vi "SynthHD_3_2a.vi"() -> ()   [LabVIEW 2017]
uses:
  Tab1.ctl
  <vilib>/Utility/file.llb/Write Delimited Spreadsheet (DBL).vi
  <vilib>/Utility/file.llb/Read Delimited Spreadsheet (DBL).vi
panel:
  in  "boot":bool=TRUE
  out "HD2":bool
  in  "CSD":bool
  out "RFOnB2":bool
  out "RFOnA2":bool
  out "Level B 2":bool
  out "Level A 2":bool
  in  "Modon":bool
  in  "Sync":bool
  out "POWER dBm B":dbl min=-100.0 max=24.0 step=1.0 format="%.2g"
  out "POWER dBm A":dbl min=-100.0 max=24.0 step=1.0 format="%.2g"
  out "RF  FREQUENCY MHz  B":dbl=1000.0 min=54.0 max=13900.0 step=1.0 format="%.7g"
  out "RF  FREQUENCY MHz A":dbl=1000.0 min=54.0 max=13900.0 step=1.0 format="%.7g"
  out "Amp Delta A -B":dbl format="%.2g"
  out "Freq Delta A-B":dbl format="%.7f"
  out "Device Under Control":string
  in  "AKNR":bool
  in  "PKNR":bool
  in  "FKNR":bool
  out "Channel":string="A"
  in  "ChSt":bool=TRUE
  out "COM Error":bool
  in  "Serial Port Select":refnum<visa-resource-name>="COM3"
  in  "stop":bool
  in  "Main Tab":T1
  in  "adn":bool
  in  "aup":bool
  in  "pdn":bool
  in  "pup":bool
  in  "fdn":bool
  in  "fup":bool
  out "Level":bool
  in  "Power Step Size":i32(ring)=3 items=["0.01dB", "0.05dB", "0.1 dB", "0.5 dB", "1.0 dB", "5.0 dB", "10.0 dB"]
  in  "RF  FREQUENCY MHz":dbl=1000.0 min=53.0 max=13999.999 step=1.0 format="%.7g"
  in  "Freqkn":i8(knob)=1 scale=1.0..20.0
  in  "Phasekn":i8(knob)=1 scale=1.0..20.0
  in  "PHASE Degrees":dbl min=0.0 max=360.0 step=1.0 format="%.2g"
  in  "POWER dBm":dbl min=-75.0 max=20.0 step=1.0 format="%.2g"
  in  "Powerkn":i8(knob)=1 scale=1.0..20.0
  in  "Frequency Step Size":i32(ring)=7 items=["0.1Hz", "1Hz", "10Hz", "100Hz", "1KHz", "10KHz", "100KHz", "1MHz", "10MHz", "100MHz", "1GHz"]
  in  "Phase Step Size":i32(ring)=6 items=["0.01 Degree", "0.05 Degree", "0.1 Degree", "0.5 Degree", "1 Degree", "5 Degree", "10 Degree", "90 Degree", "180 Degree"]
  in  "RF On":bool=TRUE
  in  "ChLock":bool
  in  "Sweep":enum32{"Linear", "List"}(tab)
  in  "Leveling":bool
  in  "Start Frequency":dbl=54.0 min=53.0 max=13999.999 step=0.001 format="%7.7f"
  in  "Step Size MHz (or %)":dbl=50.0 min=1e-07 max=23990.0 step=0.001 format="%.7f"
  in  "Stop Frequency":dbl=4000.0 min=53.0 max=13999.999 step=0.001 format="%7.7f"
  in  "Start Amplitude":dbl=22.0 min=-80.0 max=22.0 step=0.01 format="%7.2f"
  in  "Stop Amplitude":dbl=22.0 min=-80.0 max=22.0 step=0.01 format="%7.2f"
  out "Number\nof Points":u16
  out "Time per\nSweep (mS)":dbl format="%#.6g"
  in  "SwType":bool
  in  "Read Table\nFrom  CSV":bool
  in  "Save Table\nTo CSV File":bool
  in  "Table RAM to\nTable NVROM":bool
  in  "Send Table\nTo RAM":bool
  in  "Sweep Table":dbl[][](array[numeric]) format="%#.6f"
  in  "Read Table\nFrom Device":bool
  in  "sweepdiff":bool
  in  "Sweep\nOnce":bool
  in  "Sweep\nContinuously":bool
  in  "sweepdir":bool
  in  "Differential Freq":dbl=54.0 min=-13800.0 max=13800.0 step=0.001 format="%7.7f"
  in  "Step Time (mS)":dbl=4.0 min=0.1 max=10000.0 step=0.001 format="%.3f"
  out "Swpc":string
  in  "Mod Tab":enum32{"PULSE Amplitude", "AM", "FM"}(tab)
  in  "Dual Channel Mode":bool
  in  "Send Pulse\nBurst":bool
  out "Duration (uS)":dbl
  in  "Continuous\nPM":bool
  in  "# of Pulses in Burst":u16=100 min=1 max=65500 step=1 format="%#.5f"
  in  "Off Time (uS)":u32=10 min=2 max=10000000 step=1
  in  "On Time (uS)":u32=1 max=10000000 step=1
  out "Pulsech":string
  in  "Invert\nPulse":bool
  in  "Read AM":bool
  out "Samples/Cycle":u8
  in  "Save AM to ROM":bool
  out "AMch":string
  in  "AM Freq (Hz)":dbl=500.0 min=1.0 max=5000.0 step=1.0 format="%.2f"
  out "Actual Freq (Hz)":dbl
  in  "Peak Power(dBm)":dbl=15.0 min=-74.9 max=20.0 step=0.01 format="%.2f"
  in  "Minimum Power (dBm)":dbl=15.0 min=-74.9 max=20.0 step=0.01 format="%.2f"
  in  "Continuous AM":bool
  in  "Wave Shape":u8(ring) items=["Sine", "Ramp", "Triangle"]
  out "Waveform":dbl[](graph)
  in  "Linear in?":u8(ring) items=["Linear in dB", "Linear in Volts"]
  in  "AM Samples in Burst":u16=100 min=1 max=5000 step=1 format="%#.5f"
  in  "FM Rate (Hz)":u16=500 min=1 max=20000 step=1
  in  "FM Deviation (+/- Hz)":u32=500 min=10 step=1
  in  "Continuous FM":bool
  in  "FM Samples in Burst":u16=100 min=1 max=65500 step=1 format="%#.5f"
  out "FMch":string
  in  "FM Function":u8(ring) items=["Sine", "Chirp"]
  out "FM Samples / Cycle":u16
  out "Specific Instructions":string
  in  "Trigger":i32(ring) items=["No Triggers", "Full Frequency Sweep", "Single Sweep Step", "Stop All", "Digital RF On/Off", "Remove Interrupts", "Reserved 1", "Reserved 2", "Ext AM Modulation", "Ext FM Modulation"]
  out "read buffer":string
  in  "Query1":bool
  in  "Query2":bool
  in  "Query3":bool
  in  "Query4":bool
  in  "MUX Out Select":u8(ring)=6 items=["HiZ", "Vdd", "GND", "R Divider", "N Divider", "An Lock Det", "Dig Lock Det"]
  in  "PLL ICP":u8=4 max=15 step=1 format="%02d"
  out "HW Version":string
  in  "Get Phase\nLock Status":bool
  out "FW Version":string
  in  "Read\nVersion":bool
  in  "Save Settings\nto ROM":bool
  in  "Get\nTemperature":bool
  out "Temperature":string
  in  "Fundamental\nFeedback Mode":bool
  out "Lock":bool
  in  "MTLD":bool
  in  "Re-Init Settings\nto Default":bool
  in  "Reference Select":u8(ring)=1 items=["External", "Internal 27MHz", "Internal 10MHz"]
  in  "Reference (MHz)":dbl=27.0 min=5.0 max=111.0 step=0.001 format="%7.6g"
  in  "AutoCal":bool=TRUE
  in  "Channel\nSpacing":dbl=100.0 min=0.01 max=10000.0 step=0.01 format="%.2f"
  # "A"
  # "B"
  # "v3.2a"
  # "Windfreak Technologies"
  # "A"
  # "B"
  # "Tab selection dictates sweep mode"
  # "Step"
  # "Freq(MHz)"
  # "Level(dBm)"
  # "right click table for more options"
  # "Burst"
  # "Software will not respond during \"Pulse Burst\" for lower jitter."
  # "Widest FM Deviation+/- \n54-106.25MHz = 160KHz\n-212.5MHz        = 312KHz\n-425.0MHz        = 625KHz\n-850.0MHz      = 1.25MHz\n-1700MHz         = 2.5MHz\n-3400MHz            = 5MHz\n-6800MHz          = 10MHz\n-13600MHz        = 20MHz"
  # "Digital Trigger 0V to +3.3V only.\nAnalog Input 0V to 1.2V only.\nTrigger has ~35K ohm pullup\nfor both modes."
  # "Read Settings"
  # "C"
  # "Windfreak Technologies, LLC 2019"
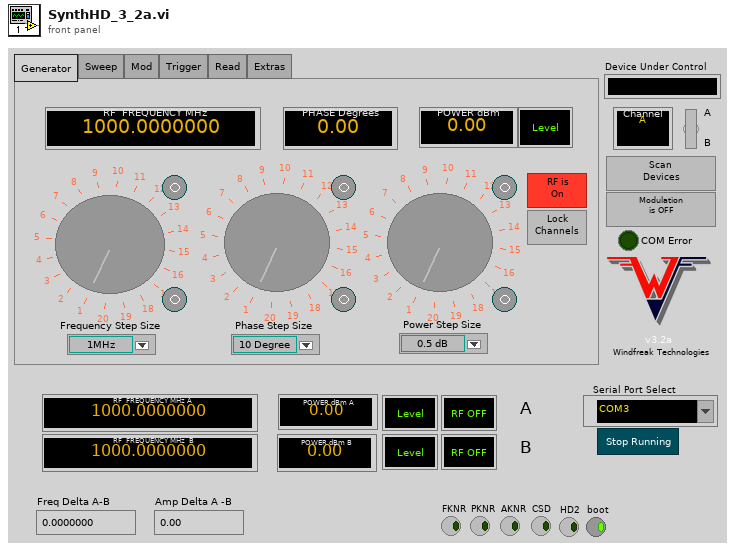
[diagram p1: front panel]
types:
  T1 = typedef "Tab1.ctl" = enum32{"Generator", "Sweep", "Mod", "Trigger", "Read", "Extras"}
  T2 = enum8{"Enabled", "Disabled", "Disabled and Grayed Out"}
  T3 = cluster{"[0]":dbl, "[1]":dbl, "[2]":dbl, "[3]":dbl, "[4]":dbl, "[5]":dbl, "[6]":dbl, "[7]":dbl, "[8]":dbl, "[9]":dbl, "[10]":dbl, "[11]":dbl, "[12]":dbl, "[13]":dbl, "[14]":dbl, "[15]":dbl, "[16]":dbl, "[17]":dbl, "[18]":dbl, "[19]":dbl, "[20]":dbl, "[21]":dbl, "[22]":dbl, "[23]":dbl, "[24]":dbl, "[25]":dbl, "[26]":dbl, "[27]":dbl, "[28]":dbl, "[29]":dbl, "[30]":dbl, "[31]":dbl, "[32]":dbl, "[33]":dbl, "[34]":dbl, "[35]":dbl, "[36]":dbl, "[37]":dbl, "[38]":dbl, "[39]":dbl, "[40]":dbl, "[41]":dbl, "[42]":dbl, "[43]":dbl, "[44]":dbl}
  T4 = typedef "LVPoint32TypeDef.ctl" = cluster{"Horizontal":i32, "Vertical":i32}
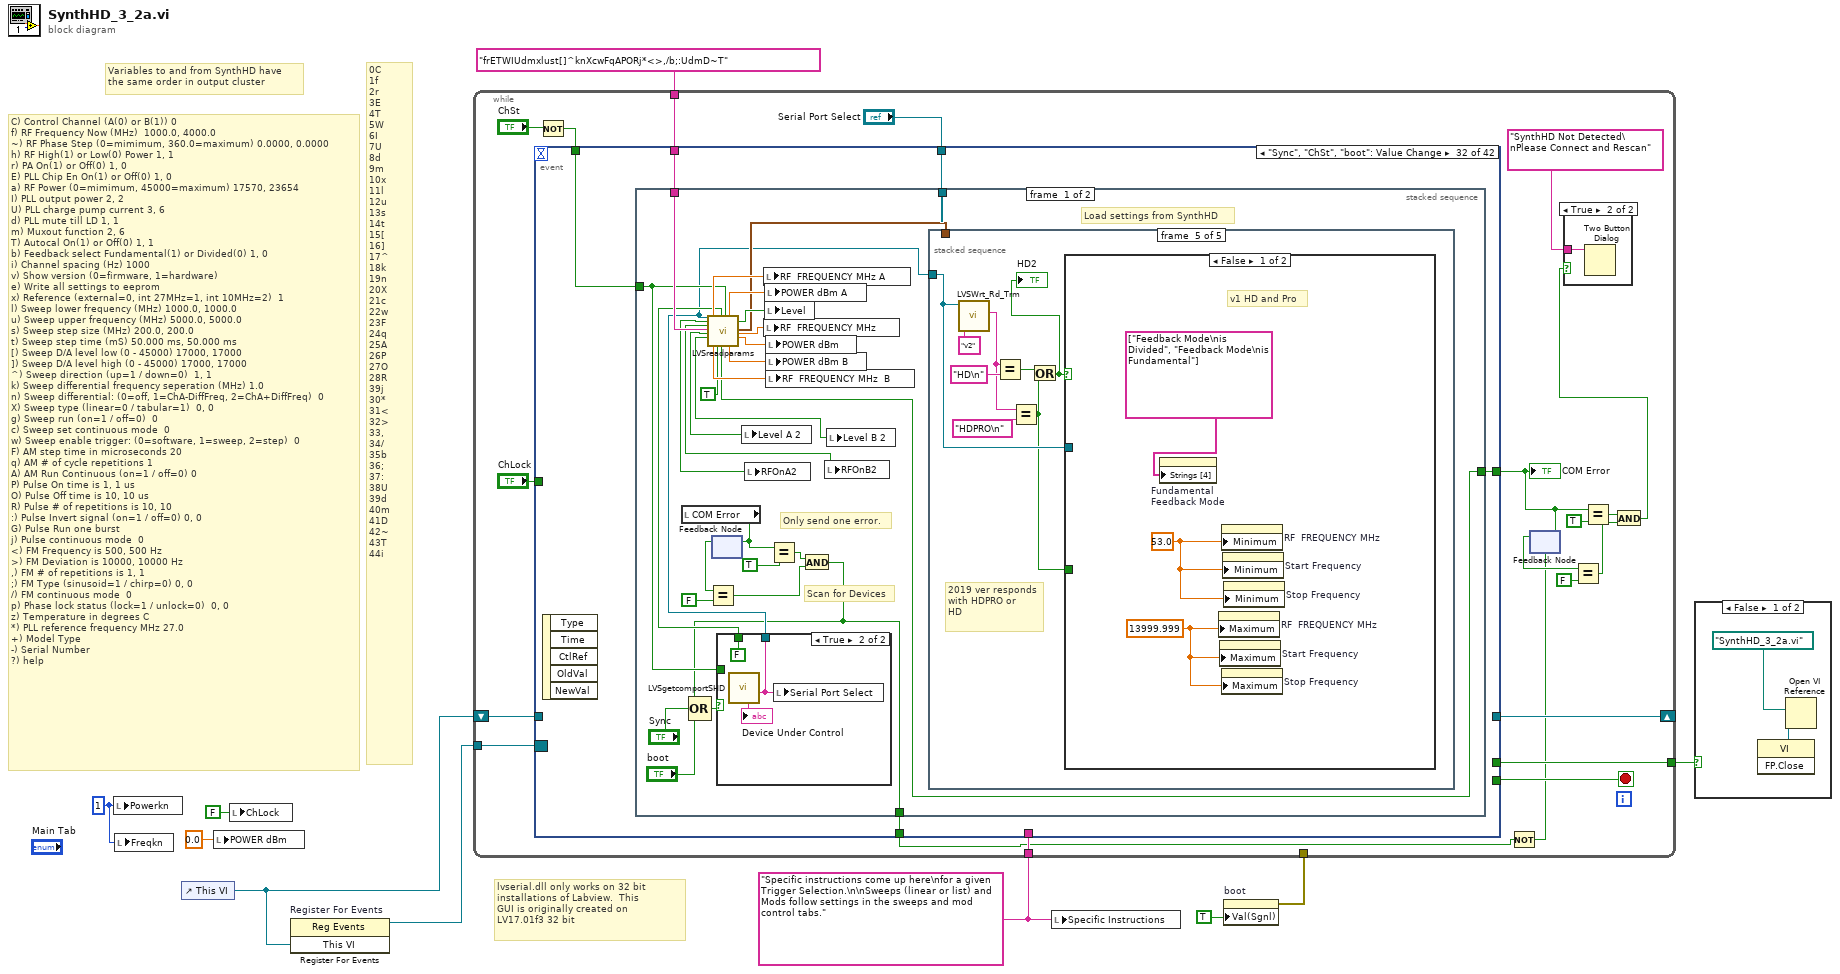
[diagram p0: block diagram]
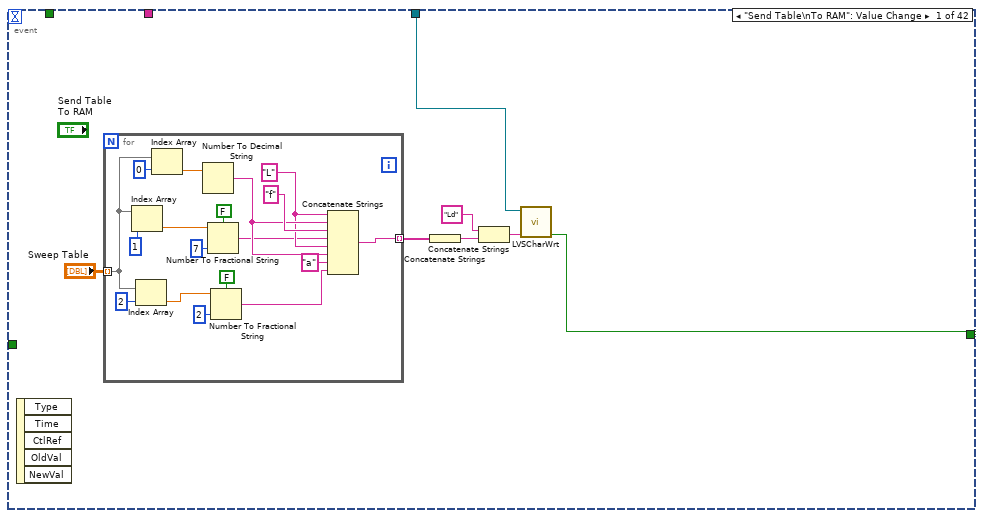
[diagram p4: hidden frame]
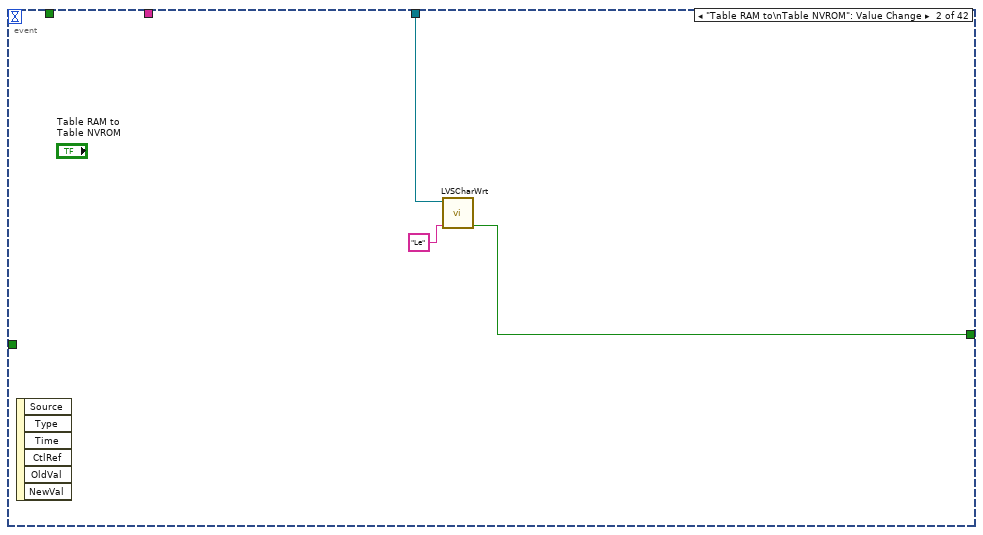
[diagram p5: hidden frame]
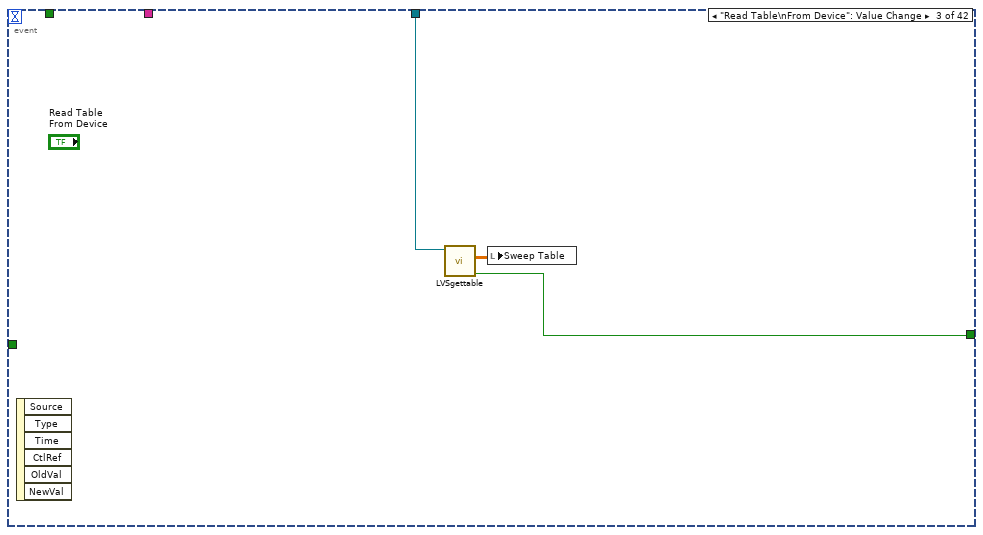
[diagram p6: hidden frame]
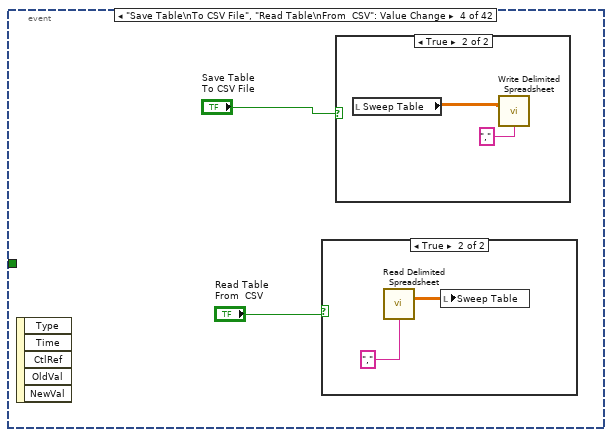
[diagram p7: hidden frame]
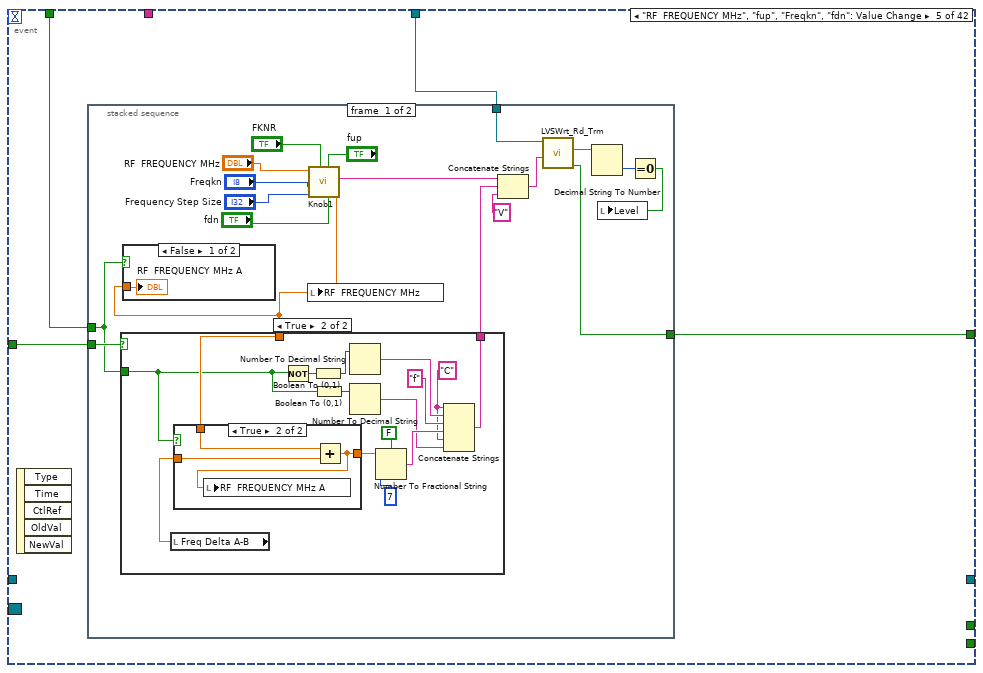
[diagram p10: hidden frame]
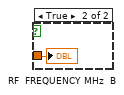
[diagram p11: hidden frame]
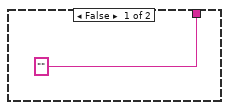
[diagram p12: hidden frame]
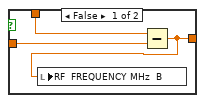
[diagram p13: hidden frame]
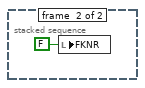
[diagram p14: hidden frame]
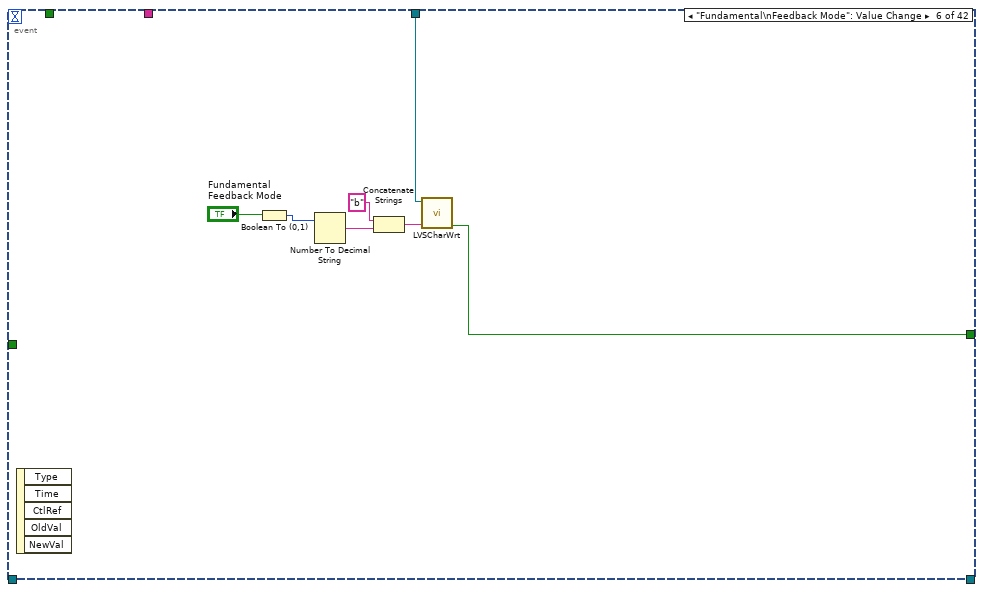
[diagram p15: hidden frame]
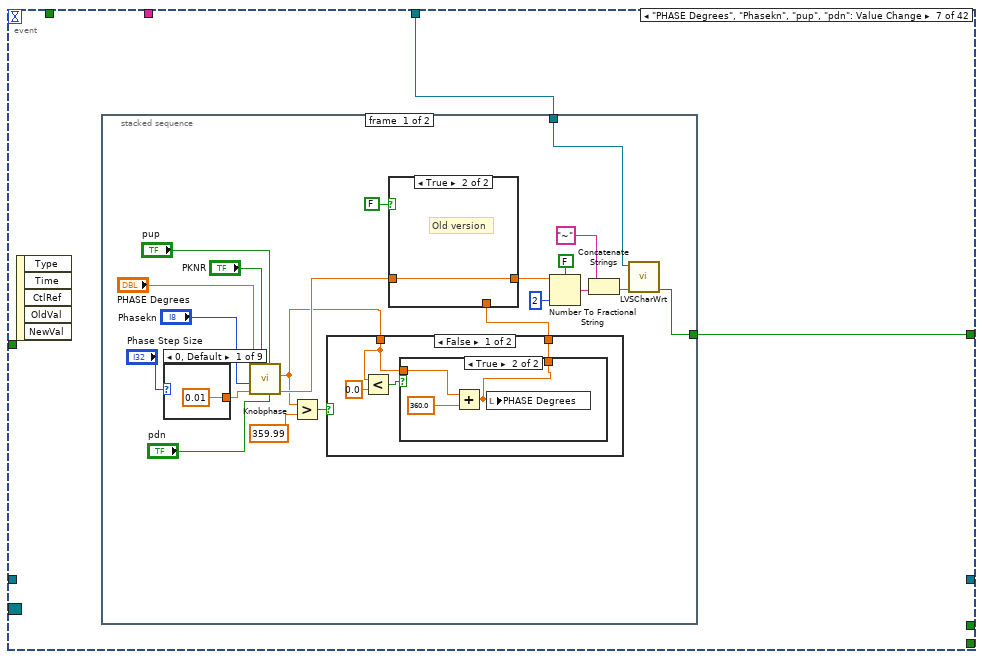
[diagram p16: hidden frame]
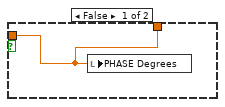
[diagram p18: hidden frame]
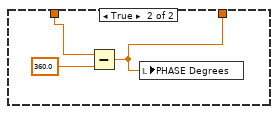
[diagram p19: hidden frame]
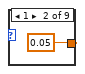
[diagram p20: hidden frame]
diagram:
  w4 = "Specific instructions come up here\nfor a given Trigger Selection.\n\nSweeps (linear or list) and Mods follow settings in the sweeps and mod control tabs." ("message")
  w8 = i8 1 ("Powerkn")
  # "lvserial.dll only works on 32 bit\ninstallations of Labview.  This\nGUI is originally created on\nLV17.01f3 32 bit"
  # "C) Control Channel (A(0) or B(1)) 0\nf) RF Frequency Now (MHz)  1000.0, 4000.0\n~) RF Phase Step (0=mimimum, 360.0=maximum) 0.0000, 0.0000\nh) RF High(1) or Low(0) Power 1, 1\nr) PA On(1) or Off(0) 1, 0\nE) PLL Chip En On(1) or Off(0) 1, 0\na) RF Power (0=mimimum, 45000=maximum) 17570, 23654\nI) PLL output power 2, 2\nU) PLL charge pump current 3, 6\nd) PLL mute till LD 1, 1\nm) Muxout function 2, 6\nT) Autocal On(1) or Off(0) 1, 1\nb) Feedback select Fundamental(1) or Divided(0) 1, 0\ni) Channel spacing (Hz) 1000\nv) Show version (0=firmware, 1=hardware)\ne) Write all settings to eeprom\nx) Reference (external=0, int 27MHz=1, int 10MHz=2)  1\nl) Sweep lower frequency (MHz) 1000.0, 1000.0\nu) Sweep upper frequency (MHz) 5000.0, 5000.0\ns) Sweep step size (MHz) 200.0, 200.0\nt) Sweep step time (mS) 50.000 ms, 50.000 ms\n[) Sweep D/A level low (0 - 45000) 17000, 17000\n]) Sweep D/A level high (0 - 45000) 17000, 17000\n^) Sweep direction (up=1 / down=0)  1, 1\nk) Sweep differential frequency seperation (MHz) 1.0\nn) Sweep differential: (0=off, 1=ChA-DiffFreq, 2=ChA+DiffFreq)  0\nX) Sweep type (linear=0 / tabular=1)  0, 0\ng) Sweep run (on=1 / off=0)  0\nc) Sweep set continuous mode  0\nw) Sweep enable trigger: (0=software, 1=sweep, 2=step)  0\nF) AM step time in microseconds 20\nq) AM # of cycle repetitions 1\nA) AM Run Continuous (on=1 / off=0) 0\nP) Pulse On time is 1, 1 us\nO) Pulse Off time is 10, 10 us\nR) Pulse # of repetitions is 10, 10\n:) Pulse Invert signal (on=1 / off=0) 0, 0\nG) Pulse Run one burst\nj) Pulse continuous mode  0\n<) FM Frequency is 500, 500 Hz\n>) FM Deviation is 10000, 10000 Hz\n,) FM # of repetitions is 1, 1\n;) FM Type (sinusoid=1 / chirp=0) 0, 0\n/) FM continuous mode  0\np) Phase lock status (lock=1 / unlock=0)  0, 0\nz) Temperature in degrees C\n*) PLL reference frequency MHz 27.0\n+) Model Type\n-) Serial Number  \n?) help"
  # "0C\n1f\n2r\n3E\n4T\n5W\n6I\n7U\n8d\n9m\n10x\n11l\n12u\n13s\n14t\n15[\n16]\n17^\n18k\n19n\n20X\n21c\n22w\n23F\n24q\n25A\n26P\n27O\n28R\n39j\n30*\n31<\n32>\n33,\n34/\n35b\n36;\n37:\n38U\n39d\n40m\n41D\n42~\n43T\n44i"
  # "Variables to and from SynthHD have \nthe same order in output cluster"
  n1 = local write "Powerkn"(w8) -> ()
  n2 = local write "Freqkn"(w8) -> ()
  n3 = control-ref of="This VI"() -> (w6:refnum<vi>)
  n4 = local write "POWER dBm"(0.0 ("Power")) -> ()
  n5 = local write "ChLock"(FALSE ("ChLock")) -> ()
  n6 = register-events "Register For Events"(w6) -> (reference out=w7:refnum<event-registration>)  [unwired: 2 in, 1 out]
  n7 = local write "Specific Instructions"(w4) -> ()
  n8 = property on="boot" class="Bool (strict)"("Val(Sgnl)"=TRUE ("boot")) -> (error out=w2:errorcluster)  [unwired: 2 in, 1 out]
  n9 = while {
    shift-right: [w27] -> _
    shift-left: w6 -> [w29]
    tunnel: w7 -> [w28]
    tunnel: [w26] -> w5
    tunnel: "frETWIUdmxlust[]^knXcwFqAPORj*<>,/b;:UdmD~T" ("var query") -> [w25]
    tunnel: w4 -> [w21]
    tunnel: w2 -> [_]
    stop <- w30 stop-if-true
    n10 = Not(x="ChSt") -> (.not. x?=w23:bool)
    n11 = event shown="[31] \"Sync\", \"ChSt\", \"boot\": Value Change" {
      selector: w28 -> [_ _ _ _ _ _ _ _ _ _ _ _ _ _ _ _ _ _ _ _ _ _ _ _ _ _ _ _ _ _ _ _ _ _ _ _ _ _ _ _ _ _]
      dyn-events: _ -> [_ _ _ _ _ _ _ _ _ _ _ _ _ _ _ _ _ _ _ _ _ _ _ _ _ _ _ _ _ _ _ _ _ _ _ _ _ _ _ _ _ _]
      timeout: _ -> [_ _ _ _ _ _ _ _ _ _ _ _ _ _ _ _ _ _ _ _ _ _ _ _ _ _ _ _ _ _ _ _ _ _ _ _ _ _ _ _ _ _]
      tunnel: "Serial Port Select" -> [w33 w59 w62 _ w73 w118 w125 w173 w238 _ w266 w317 w327 w344 w362 w387 w406 w409 w439 w442 w461 w471 w474 w481 w486 w495 w498 w516 w523 w530 w541 w552 w712 w720 w748 w766 _ _ _ _ w858 w870]
      tunnel: [_ _ _ _ _ _ _ _ _ _ _ _ _ _ _ _ _ _ _ _ _ _ _ _ _ _ _ _ _ _ _ _ _ _ _ _ _ "stop" w854 _ _ _] -> w30
      tunnel: w29 -> [_ _ _ _ _ _ _ _ _ _ _ _ _ _ _ _ _ _ _ _ _ _ _ _ _ _ _ _ _ _ _ _ _ _ _ _ _ _ w853 _ _ _]
      tunnel: [_ _ _ _ _ _ _ _ _ _ _ _ _ _ _ _ _ _ _ _ _ _ _ _ _ _ _ _ _ _ _ _ _ _ _ _ _ _ w853 _ _ _] -> w27
      tunnel: [_ _ _ _ _ _ _ _ _ _ _ _ _ _ _ _ _ _ _ _ _ _ _ _ _ _ _ _ _ _ _ _ _ _ _ _ _ "stop" _ _ _ _] -> w26
      tunnel: w25 -> [_ _ _ _ _ _ _ _ _ _ _ _ _ _ _ _ _ _ _ _ _ _ _ _ _ _ _ _ _ _ _ w553 _ _ _ _ _ _ _ _ _ _]
      tunnel: w23 -> [_ _ _ _ w72 _ _ w172 w241 _ _ _ _ _ w363 w394 _ w420 _ w449 _ _ _ _ _ _ _ _ _ _ _ w551 _ _ w752 _ _ _ _ _ _ _]
      tunnel: "ChLock" -> [_ _ _ _ w71 _ _ w171 _ _ _ _ _ _ _ _ _ _ _ _ _ _ _ _ _ _ _ _ _ _ _ _ _ _ _ _ _ _ _ _ _ _]
      tunnel: w21 -> [_ _ _ _ _ _ _ _ _ _ _ _ w329 _ _ _ _ _ _ _ _ _ _ _ _ _ _ _ _ _ _ _ _ _ _ _ _ _ _ _ _ _]
      tunnel: [w34 w58 w61 _ w70 w117 w124 w170 w237 _ w263 w316 w326 w343 w361 w386 w405 w408 w437 w440 w459 w470 w473 w479 w482 w492 w496 w515 w521 w528 w540 w550 w711 w719 w747 w765 w785 _ _ _ w857 _] -> w15
      tunnel: [_ _ _ _ _ _ _ _ _ _ _ _ _ _ _ _ _ _ _ _ _ _ _ _ _ _ _ _ _ _ _ w549 _ _ _ _ _ _ _ _ _ _] -> w12
      event "Send Table\nTo RAM": Value Change {
        n12 = event-data() -> ()  [unwired: 1 in, 5 out]
        n13 = for {
          tunnel: "Sweep Table" -> [w46] mode=indexing
          tunnel: [w52] -> w36 mode=indexing
          w49 = "L" ("string")
          n14 = Index Array(array=w46, index=1) -> (element=w45:dbl)
          n15 = Index Array(array=w46, index=2) -> (element=w41:dbl)
          n16 = Index Array(array=w46, index=0) -> (element=w50:dbl)
          n17 = Number To Decimal String(number=w50) -> (decimal integer string=w53:string)  [unwired: 1 in]
          n18 = Number To Fractional String(use system decimal point (T)=FALSE, number=w45, precision (6)=i16 7) -> (F-format string=w48:string)  [unwired: 1 in]
          n19 = Number To Fractional String(use system decimal point (T)=FALSE, number=w41, precision (6)=i16 2) -> (F-format string=w40:string)  [unwired: 1 in]
          n20 = Concatenate Strings(w49, w53, "f" ("string"), w48, w49, w53, "a" ("string"), w40) -> (w52:string)
        }
        n21 = Concatenate Strings(w36) -> (w38:string)
        n22 = Concatenate Strings("Ld" ("string"), w38) -> (w35:string)
        n23 = call "LVSCharWrt.vi"("String In"=w35, "COM Port"=w33) -> ("ComError"=w34:bool)  [unwired: 9 in]
      }
      event "Table RAM to\nTable NVROM": Value Change {
        n24 = event-data() -> ()  [unwired: 1 in, 6 out]
        n25 = call "LVSCharWrt.vi"("String In"="Le" ("write buffer"), "COM Port"=w59) -> ("ComError"=w58:bool)  [unwired: 9 in]
      }
      event "Read Table\nFrom Device": Value Change {
        n26 = event-data() -> ()  [unwired: 1 in, 6 out]
        n27 = call "LVSgettable.vi"("Serial Port Select"=w62) -> ("COM Error"=w61:bool, "Sweep Table"=w63:dbl[][])  [unwired: 9 in]
        n28 = local write "Sweep Table"(w63) -> ()
      }
      event "Save Table\nTo CSV File", "Read Table\nFrom  CSV": Value Change {
        n29 = event-data() -> ()  [unwired: 1 in, 5 out]
        n30 = case shown="True" "Read Table\nFrom  CSV" {
          frame False {
          }
          frame True {
            n31 = call-poly <vilib>:"Read Delimited Spreadsheet.vi"("delimiter (\\t)"="," ("delimiter (\\t)")) -> ("all rows"=w67:dbl[][])  [unwired: 9 in, 5 out]
            n32 = local write "Sweep Table"(w67) -> ()
          }
        }
        n33 = case shown="True" "Save Table\nTo CSV File" {
          frame False {
          }
          frame True {
            n34 = local read "Sweep Table"() -> (w69:dbl[][])
            n35 = call-poly <vilib>:"Write Delimited Spreadsheet.vi"("2D data"=w69, "delimiter (\\t)"="," ("delimiter (\\t)")) -> ()  [unwired: 12 in, 2 out]
          }
        }
      }
      event "RF  FREQUENCY MHz", "fup", "Freqkn", "fdn": Value Change {
        n36 = event-data() -> ()  [unwired: 1 in, 5 out]
        n37 = stacked-sequence {
          tunnel: w73 -> [w77 _]
          tunnel: w72 -> [w82 _]
          tunnel: w71 -> [w84 _]
          tunnel: [w75 _] -> w70
          frame #0 {
            n38 = call "Knob1.vi"("Freqin"="RF  FREQUENCY MHz", "Knob"="Freqkn", "Frequency Step Size"="Frequency Step Size", "Reset"="FKNR", "fup"="fup", "fdn"="fdn") -> ("freqcommand"=w89:string, "freqout"=w81:dbl)  [unwired: 3 in]
            n39 = case shown="True" w84 {
              tunnel: ["" ("string") w109] -> w83
              tunnel: w81 -> [_ w100]
              tunnel: w82 -> [_ w97]
              frame False {
              }
              frame True {
                w96 = "C" ("string")
                n40 = local read "Freq Delta A-B"() -> (w102:dbl)
                n41 = case shown="True" w97 {
                  tunnel: w100 -> [w111 w115]
                  tunnel: [w110 w113] -> w99
                  tunnel: w102 -> [w112 w114]
                  frame False {
                    n42 = Subtract(x=w111, y=w112) -> (x-y=w110:dbl)
                    n43 = local write "RF  FREQUENCY MHz  B"(w110) -> ()
                  }
                  frame True {
                    n44 = Add(x=w115, y=w114) -> (x+y=w113:dbl)
                    n45 = local write "RF  FREQUENCY MHz A"(w113) -> ()
                  }
                }
                n46 = Not(x=w97) -> (.not. x?=w98:bool)
                n47 = Boolean To (0,1)(Boolean=w98) -> (0, 1=w104:i16)
                n48 = Boolean To (0,1)(Boolean=w97) -> (0, 1=w103:i16)
                n49 = Number To Decimal String(number=w104) -> (decimal integer string=w108:string)  [unwired: 1 in]
                n50 = Number To Decimal String(number=w103) -> (decimal integer string=w95:string)  [unwired: 1 in]
                n51 = Number To Fractional String(use system decimal point (T)=FALSE, number=w99, precision (6)=i16 7) -> (F-format string=w105:string)  [unwired: 1 in]
                n52 = Concatenate Strings(w96, w108, "f" ("string"), w105, w96, w95) -> (w109:string)
              }
            }
            n53 = case shown="False" w82 {
              tunnel: w81 -> [w92 w93]
              frame False {
                "RF  FREQUENCY MHz A" <- w92
              }
              frame True {
                "RF  FREQUENCY MHz  B" <- w93
              }
            }
            n54 = local write "RF  FREQUENCY MHz"(w81) -> ()
            n55 = Concatenate Strings(w89, w83, "V" ("string")) -> (w76:string)
            n56 = call "LVSWrt_Rd_Trm.vi"("WriteBuf"=w76, "COM Port"=w77) -> ("ComError"=w75:bool, "string read"=w74:string)  [unwired: 8 in]
            n57 = Decimal String To Number(string=w74) -> (number=w78:i32)  [unwired: 2 in, 1 out]
            n58 = Equal To 0?(x=w78) -> (x = 0?=w79:bool)
            n59 = local write "Level"(w79) -> ()
          }
          frame #1 {
            n60 = local write "FKNR"(FALSE ("Reset")) -> ()
          }
        }
      }
      event "Fundamental\nFeedback Mode": Value Change {
        n61 = event-data() -> ()  [unwired: 1 in, 5 out]
        n62 = Boolean To (0,1)(Boolean="Fundamental\nFeedback Mode") -> (0, 1=w122:i16)
        n63 = Number To Decimal String(number=w122) -> (decimal integer string=w121:string)  [unwired: 1 in]
        n64 = Concatenate Strings("b" ("element"), w121) -> (w119:string)
        n65 = call "LVSCharWrt.vi"("String In"=w119, "COM Port"=w118) -> ("ComError"=w117:bool)  [unwired: 9 in]
      }
      event "PHASE Degrees", "Phasekn", "pup", "pdn": Value Change {
        n66 = event-data() -> ()  [unwired: 1 in, 5 out]
        n67 = stacked-sequence {
          tunnel: w125 -> [w127 _]
          tunnel: [w126 _] -> w124
          frame #0 {
            n68 = case shown="0, Default" "Phase Step Size" {
              tunnel: [0.01 0.05 0.1 0.5 1.0 5.0 10.0 90.0 180.0] -> w136
              frame 0, Default {
              }
              frame 1 {
              }
              frame 2 {
              }
              frame 3 {
              }
              frame 4 {
              }
              frame 5 {
              }
              frame 6 {
              }
              frame 7 {
              }
              frame 8 {
              }
            }
            n69 = call "Knobphase.vi"("Freqin"="PHASE Degrees", "Knob"="Phasekn", "Step Size"=w136, "Reset"="PKNR", "pup"="pup", "pdn"="pdn") -> ("Freqout"=w131:dbl, "Phase Pr Out"=w133:dbl)  [unwired: 3 in]
            n70 = Greater?(x=w131, y=359.99) -> (0:w138:bool)
            n71 = case shown="False" w138 {
              tunnel: w131 -> [w150 w158]
              tunnel: [w149 w157] -> w129
              frame False {
                n72 = Less?(x=w150, y=0.0) -> (x < y?=w151:bool)
                n73 = case shown="True" w151 {
                  tunnel: w150 -> [w153 w154]
                  tunnel: [w153 w156] -> w149
                  frame False {
                    n74 = local write "PHASE Degrees"(w153) -> ()
                  }
                  frame True {
                    n75 = Add(x=w154, y=360.0 ("Phase Degrees")) -> (x+y=w156:dbl)
                    n76 = local write "PHASE Degrees"(w156) -> ()
                  }
                }
              }
              frame True {
                n77 = Subtract(x=w158, y=360.0 ("Phase Degrees")) -> (x-y=w157:dbl)
                n78 = local write "PHASE Degrees"(w157) -> ()
              }
            }
            n79 = case shown="True" FALSE {
              tunnel: w133 -> [_ w148]
              tunnel: [w147 w148] -> w132
              tunnel: w129 -> [w147 _]
              frame False {
                # "New version"
              }
              frame True {
                # "Old version"
              }
            }
            n80 = Number To Fractional String(use system decimal point (T)=FALSE, number=w132, precision (6)=i16 2) -> (F-format string=w144:string)  [unwired: 1 in]
            n81 = Concatenate Strings("~" ("element"), w144) -> (w128:string)
            n82 = call "LVSCharWrt.vi"("String In"=w128, "COM Port"=w127) -> ("ComError"=w126:bool)  [unwired: 9 in]
          }
          frame #1 {
            n83 = local write "PKNR"(FALSE ("PKNR")) -> ()
          }
        }
      }
      event "Powerkn", "POWER dBm", "aup", "adn": Value Change {
        n84 = event-data() -> ()  [unwired: 1 in, 5 out]
        n85 = stacked-sequence {
          tunnel: w173 -> [w178 _]
          tunnel: w172 -> [w179 _]
          tunnel: w171 -> [w187 _]
          tunnel: [w174 _] -> w170
          frame #0 {
            # "Sweep Leveling"
            # "write to VGA"
            n86 = case shown="3" "Power Step Size" {
              tunnel: [0.01 0.05 0.1 0.5 1.0 5.0 10.0] -> w193
              frame 0, Default {
              }
              frame 1 {
              }
              frame 2 {
              }
              frame 3 {
              }
              frame 4 {
              }
              frame 5 {
              }
              frame 6 {
              }
            }
            n87 = call "Knob3.vi"("PwrIn"="POWER dBm", "Knob"="Powerkn", "Step Size"=w193, "Reset"="AKNR", "aup"="aup", "adn"="adn") -> ("PwrSet"=w182:string, "PwrOut"=w183:dbl)  [unwired: 3 in]
            n88 = case shown="True" w187 {
              tunnel: ["" ("string") w222] -> w186
              tunnel: w179 -> [_ w215]
              tunnel: w183 -> [_ w218]
              frame False {
              }
              frame True {
                w210 = "C" ("string")
                n89 = local read "Amp Delta A -B"() -> (w219:dbl)
                n90 = case shown="True" w215 {
                  tunnel: [w223 w226] -> w214
                  tunnel: w219 -> [w225 w228]
                  tunnel: w218 -> [w224 w227]
                  frame False {
                    n91 = Subtract(x=w224, y=w225) -> (x-y=w223:dbl)
                    n92 = local write "POWER dBm B"(w223) -> ()
                  }
                  frame True {
                    n93 = Add(x=w227, y=w228) -> (x+y=w226:dbl)
                    n94 = local write "POWER dBm A"(w226) -> ()
                  }
                }
                n95 = Not(x=w215) -> (.not. x?=w216:bool)
                n96 = Boolean To (0,1)(Boolean=w216) -> (0, 1=w221:i16)
                n97 = Boolean To (0,1)(Boolean=w215) -> (0, 1=w220:i16)
                n98 = Number To Decimal String(number=w221) -> (decimal integer string=w209:string)  [unwired: 1 in]
                n99 = Number To Decimal String(number=w220) -> (decimal integer string=w217:string)  [unwired: 1 in]
                n100 = Number To Fractional String(use system decimal point (T)=FALSE, number=w214, precision (6)=i16 2) -> (F-format string=w211:string)  [unwired: 1 in]
                n101 = Concatenate Strings(w210, w209, "W" ("string"), w211, w210, w217) -> (w222:string)
              }
            }
            n102 = case shown="True" w179 {
              tunnel: w183 -> [w205 w206]
              frame False {
                "POWER dBm A" <- w205
              }
              frame True {
                "POWER dBm B" <- w206
              }
            }
            n103 = local write "POWER dBm"(w183) -> ()
            n104 = local read "Leveling"() -> (w185:bool)
            n105 = case shown="True" w185 {
              tunnel: ["" ("string") w199] -> w184
              tunnel: w182 -> [_ w203]
              tunnel: w183 -> [_ w198]
              frame False {
              }
              frame True {
                n106 = String Subset(string=w203, offset (0)=1) -> (substring=w201:string)  [unwired: 1 in]
                n107 = local write "Start Amplitude"(w198) -> ()
                n108 = local write "Stop Amplitude"(w198) -> ()
                n109 = Concatenate Strings("[" ("string"), w201, "]" ("string"), w201) -> (w199:string)
              }
            }
            n110 = Concatenate Strings(w182, w186, w184, "V" ("string")) -> (w177:string)
            n111 = call "LVSWrt_Rd_Trm.vi"("WriteBuf"=w177, "COM Port"=w178) -> ("ComError"=w174:bool, "string read"=w176:string)  [unwired: 8 in]
            n112 = Decimal String To Number(string=w176) -> (number=w180:i32)  [unwired: 2 in, 1 out]
            n113 = Equal To 0?(x=w180) -> (x = 0?=w175:bool)
            "Level" <- w175
            n114 = case shown="True" w179 {
              tunnel: w175 -> [w195 w196]
              frame False {
                "Level A 2" <- w195
              }
              frame True {
                "Level B 2" <- w196
              }
            }
          }
          frame #1 {
            n115 = local write "AKNR"(FALSE ("AKNR")) -> ()
          }
        }
      }
      event "RF On": Value Change {
        # "Turn RF off and on"
        n116 = event-data() -> ()  [unwired: 1 in, 5 out]
        n117 = Boolean To (0,1)(Boolean="RF On") -> (0, 1=w244:i16)
        n118 = Number To Decimal String(number=w244) -> (decimal integer string=w243:string)  [unwired: 1 in]
        n119 = case shown="True" w241 {
          tunnel: "RF On" -> [w246 w247]
          frame False {
            "RFOnA2" <- w246
          }
          frame True {
            "RFOnB2" <- w247
          }
        }
        n120 = Concatenate Strings("E" ("element"), w243, "r" ("string"), w243) -> (w239:string)
        n121 = call "LVSCharWrt.vi"("String In"=w239, "COM Port"=w238) -> ("ComError"=w237:bool)  [unwired: 9 in]
      }
      event "ChLock": Value Change {
        n122 = event-data() -> ()  [unwired: 1 in, 5 out]
        n123 = local read "RF  FREQUENCY MHz  B"() -> (w253:dbl)
        n124 = local read "RF  FREQUENCY MHz A"() -> (w252:dbl)
        n125 = local read "POWER dBm A"() -> (w249:dbl)
        n126 = local read "POWER dBm B"() -> (w248:dbl)
        n127 = Subtract(x=w252, y=w253) -> (x-y=→"Freq Delta A-B":dbl)
        n128 = Subtract(x=w249, y=w248) -> (x-y=→"Amp Delta A -B":dbl)
      }
      event "Start Frequency", "Stop Frequency", "Step Time (mS)", "Step Size MHz (or %)", "Start Amplitude", "Stop Amplitude", "Leveling", "sweepdiff", "sweepdir", "Differential Freq", "AM Samples in Burst", "SwType", "Sweep": Value Change {
        w271 = i16 7 ("precision (6)")
        w272 = FALSE ("use system decimal point (T)")
        # "Set up Sweep"
        n129 = event-data() -> ()  [unwired: 1 in, 5 out]
        n130 = case shown="True" "Leveling" {
          tunnel: ["Start Amplitude" w315] -> w269
          tunnel: ["Stop Amplitude" w315] -> w270
          frame False {
            w311 = T2."Enabled" ("Disabled")
            n131 = property on="Start Amplitude" class="DigNum (strict)"("DisabledEnum"=w311) -> ()  [unwired: 2 in, 2 out]
            n132 = property on="Stop Amplitude" class="DigNum (strict)"("DisabledEnum"=w311) -> ()  [unwired: 2 in, 2 out]
          }
          frame True {
            w314 = T2."Disabled and Grayed Out" ("Disabled")
            n133 = local read "POWER dBm"() -> (w315:dbl)
            n134 = local write "Start Amplitude"(w315) -> ()
            n135 = local write "Stop Amplitude"(w315) -> ()
            n136 = property on="Start Amplitude" class="DigNum (strict)"("DisabledEnum"=w314) -> ()  [unwired: 2 in, 2 out]
            n137 = property on="Stop Amplitude" class="DigNum (strict)"("DisabledEnum"=w314) -> ()  [unwired: 2 in, 2 out]
          }
        }
        n138 = Subtract(x="Stop Frequency", y="Start Frequency") -> (x-y=w290:dbl)
        n139 = Divide(x=w290, y="Step Size MHz (or %)") -> (x/y=w289:dbl)
        "Number\nof Points" <- w289
        n140 = Multiply(x="Step Time (mS)", y=w289) -> (x*y=→"Time per\nSweep (mS)":dbl)
        n141 = Number To Fractional String(use system decimal point (T)=w272, number="Step Size MHz (or %)", precision (6)=w271) -> (F-format string=w293:string)  [unwired: 1 in]
        n142 = Number To Fractional String(use system decimal point (T)=w272, number="Step Time (mS)", precision (6)=w271) -> (F-format string=w291:string)  [unwired: 1 in]
        n143 = Number To Fractional String(use system decimal point (T)=w272, number="Start Frequency", precision (6)=w271) -> (F-format string=w298:string)  [unwired: 1 in]
        n144 = Number To Fractional String(use system decimal point (T)=w272, number="Stop Frequency", precision (6)=w271) -> (F-format string=w297:string)  [unwired: 1 in]
        n145 = Number To Fractional String(use system decimal point (T)=w272, number=w269, precision (6)=w271) -> (F-format string=w265:string)  [unwired: 1 in]
        n146 = Number To Fractional String(use system decimal point (T)=w272, number=w270, precision (6)=w271) -> (F-format string=w264:string)  [unwired: 1 in]
        n147 = property on="Stop Frequency" class="DigNum (strict)"("Minimum"="Start Frequency") -> ()  [unwired: 2 in, 2 out]
        n148 = property on="Start Frequency" class="DigNum (strict)"("Maximum"="Stop Frequency") -> ()  [unwired: 2 in, 2 out]
        n149 = Not(x="sweepdir") -> (.not. x?=w275:bool)
        n150 = Boolean To (0,1)(Boolean=w275) -> (0, 1=w280:i16)
        n151 = Number To Decimal String(number="AM Samples in Burst") -> (decimal integer string=w261:string)  [unwired: 1 in]
        n152 = Number To Decimal String(number=w280) -> (decimal integer string=w279:string)  [unwired: 1 in]
        n153 = Absolute Value(x="Differential Freq") -> (abs(x)=w278:dbl)
        n154 = Number To Fractional String(use system decimal point (T)=FALSE, number=w278, precision (6)=i16 7) -> (F-format string=w259:string)  [unwired: 1 in]
        n155 = case shown="\"Linear\", Default" "Sweep" {
          tunnel: [w299 "X1" ("element")] -> w256
          frame "Linear", Default {
            n156 = case shown="False" "SwType" {
              tunnel: ["X0" ("element") "X2" ("element")] -> w299
              frame False {
              }
              frame True {
              }
            }
          }
          frame "List" {
          }
        }
        n157 = case shown="True" "sweepdiff" {
          tunnel: ["n0" ("element") w305] -> w258
          tunnel: "Differential Freq" -> [_ w307]
          frame False {
          }
          frame True {
            n158 = Greater?(x=w307, y=0.0) -> (0:w306:bool)
            n159 = case shown="False" w306 {
              tunnel: ["n1" ("element") "n2" ("element")] -> w305
              frame False {
              }
              frame True {
              }
            }
          }
        }
        n160 = Concatenate Strings("l" ("element"), w298, "u" ("element"), w297, "s" ("element"), w293, "t" ("element"), w291, "[" ("element"), w265, "]" ("element"), w264, "^" ("element"), w279, "q" ("element"), w261, "k" ("element"), w259, w258, w256) -> (w267:string)
        n161 = call "LVSCharWrt.vi"("String In"=w267, "COM Port"=w266) -> ("ComError"=w263:bool)  [unwired: 9 in]
      }
      event "AutoCal": Value Change {
        n162 = event-data() -> ()  [unwired: 1 in, 6 out]
        n163 = Boolean To (0,1)(Boolean="AutoCal") -> (0, 1=w322:i16)
        n164 = Number To Decimal String(number=w322) -> (decimal integer string=w321:string)  [unwired: 1 in]
        n165 = case shown="False" "AutoCal" {
          tunnel: [0.3 ("Data Entry Limits:Minimum") 3.0 ("Data Entry Limits:Minimum")] -> w320
          frame False {
          }
          frame True {
          }
        }
        n166 = Concatenate Strings("T" ("element"), w321) -> (w318:string)
        n167 = property on="Step Time (mS)" class="DigNum (strict)"("Minimum"=w320) -> ()  [unwired: 2 in, 2 out]
        n168 = call "LVSCharWrt.vi"("String In"=w318, "COM Port"=w317) -> ("ComError"=w316:bool)  [unwired: 9 in]
      }
      event "Trigger": Value Change {
        n169 = event-data() -> ()  [unwired: 1 in, 5 out]
        n170 = case shown="9" "Trigger" {
          tunnel: [w334 "One full sweep happens after pulling down\nthe trigger signal.  It is level sensitive so\nholding down the signal repeats the sweep.\nBring high before the end of the sweep to\navoid another sweep." ("message") "Sweep Step Trigger will trigger one step in\na linear sweep or list sweep when pulled low.\nUse Step Time to debounce and make sure\nstep time is longer than your trigger pulse\nduration to avoid two steps in one pulse." ("message") "Stop All puts a \"do nothing\" hold on the\nSynthHD operating system.  It only responds\nto the Trigger and to USB.  This allows you to\ntrigger bursts of pulses or other modulations." ("message") "Quickly mutes RF power when low.  A high\nlevel restores RF power to the GUI setting." ("message") "Remove interrupts reduces jitter in modulations\nthat are timing critical.  When Trigger is pulled low\nRF is ON and Interrupts are off.  When Trigger is high\nRF is OFF and the SynthHD will respond to USB commands." ("message") "External AM Modulation is driven through the\nTrigger connector and responds to analog voltages\nbetween 0 and 1.2V.  It responds to setting stored in the\nAM look up table and cycles through each sample.  For\nbest performance set the AM frequency to 1Hz which gives\nthe maximum of 100 samples.  Set the wave shape to RAMP\nand select whether you want the response linear in dB or Volts.\n0V input will correspond with the Minimum Power setting\nand 1.2V will drive to the Peak Power setting with 100 steps\nin between.  Sample rate is roughly 22uS." ("message") "External FM Modulation is driven through the\nTrigger connector and responds to analog voltages\nbetween 0 and 1.2V.  It responds to setting stored in the\nFM control tab and cycles through each sample it creates.  For\nbest performance set the FM frequency to 1Hz which gives\nthe maximum of 100 samples.  Set the wave shape to CHIRP.\n0V input will correspond with the (neg) FM Deviation setting\nand 1.2V will drive to the (pos) Deviation setting with\n100 steps in between.  Sample rate is roughly 22uS." ("message")] -> w330
          tunnel: w329 -> [w334 _ _ _ _ _ _ _]
          frame 0, Default {
          }
          frame 1 {
          }
          frame 2 {
          }
          frame 3 {
          }
          frame 4 {
          }
          frame 5 {
            n171 = One Button Dialog(message="THIS MODE BLOCKS USB COMMUNICATIONS.\nClicking any controls while in this mode\n(with the Trigger connector pulled to ground)\nwill cause the software to lock up.  Exit this\nmode or disconnect everything from the Trigger\n connector before resuming normal operation.") -> ()  [unwired: 1 in, 1 out]
          }
          frame 8 {
          }
          frame 9 {
          }
        }
        "Specific Instructions" <- w330
        n172 = Number To Decimal String(number="Trigger") -> (decimal integer string=w332:string)  [unwired: 1 in]
        n173 = Concatenate Strings("w" ("element"), w332) -> (w328:string)
        n174 = call "LVSCharWrt.vi"("String In"=w328, "COM Port"=w327) -> ("ComError"=w326:bool)  [unwired: 9 in]
      }
      event "On Time (uS)", "Off Time (uS)", "# of Pulses in Burst", "Invert\nPulse": Value Change {
        # "Pulse Modulation"
        n175 = event-data() -> ()  [unwired: 1 in, 5 out]
        n176 = Add(x="On Time (uS)", y="Off Time (uS)") -> (x+y=w360:u32)
        n177 = Number To Decimal String(number="On Time (uS)") -> (decimal integer string=w356:string)  [unwired: 1 in]
        n178 = Number To Decimal String(number="Off Time (uS)") -> (decimal integer string=w357:string)  [unwired: 1 in]
        n179 = Number To Decimal String(number="# of Pulses in Burst") -> (decimal integer string=w358:string)  [unwired: 1 in]
        n180 = Multiply(x=w360, y="# of Pulses in Burst") -> (x*y=→"Duration (uS)":u32)
        n181 = Boolean To (0,1)(Boolean="Invert\nPulse") -> (0, 1=w349:i16)
        n182 = Number To Decimal String(number=w349) -> (decimal integer string=w347:string)  [unwired: 1 in]
        n183 = Concatenate Strings(":" ("string"), w347, "P" ("string"), w356, "O" ("string"), w357, "R" ("string"), w358) -> (w345:string)
        n184 = call "LVSCharWrt.vi"("String In"=w345, "COM Port"=w344) -> ("ComError"=w343:bool)  [unwired: 9 in]
      }
      event "Mod Tab": Value Change {
        n185 = event-data() -> ()  [unwired: 1 in, 5 out]
        n186 = local read "Modon"() -> (w364:bool)
        n187 = case shown="False" w364 {
          tunnel: w362 -> [w367 _]
          tunnel: w363 -> [w380 _]
          tunnel: [w365 FALSE ("ComError")] -> w361
          frame False {
            w381 = "C" ("string")
            w370 = "h1" ("write buffer")
            n188 = local read "RF  FREQUENCY MHz"() -> (w383:dbl)
            n189 = local read "POWER dBm"() -> (w375:dbl)
            n190 = Boolean To (0,1)(Boolean=w380) -> (0, 1=w382:i16)
            n191 = Not(x=w380) -> (.not. x?=w378:bool)
            n192 = Number To Decimal String(number=w382) -> (decimal integer string=w376:string)  [unwired: 1 in]
            n193 = Boolean To (0,1)(Boolean=w378) -> (0, 1=w379:i16)
            n194 = Number To Fractional String(use system decimal point (T)=FALSE, number=w375, precision (6)=i16 2) -> (F-format string=w368:string)  [unwired: 1 in]
            n195 = Number To Decimal String(number=w379) -> (decimal integer string=w377:string)  [unwired: 1 in]
            n196 = Number To Fractional String(use system decimal point (T)=FALSE, number=w383) -> (F-format string=w371:string)  [unwired: 2 in]
            n197 = Concatenate Strings("f" ("string"), w371, w370, "W" ("string"), w368, w381, w377, w370, w381, w376) -> (w366:string)
            n198 = call "LVSCharWrt.vi"("String In"=w366, "COM Port"=w367) -> ("ComError"=w365:bool)  [unwired: 9 in]
          }
          frame True {
          }
        }
      }
      event "Sweep\nContinuously": Value Change {
        # "Sweep Continuously"
        n199 = event-data() -> ()  [unwired: 1 in, 5 out]
        n200 = local read "Continuous AM"() -> (w390:bool)
        n201 = local read "Continuous\nPM"() -> (w392:bool)
        n202 = local read "Continuous FM"() -> (w391:bool)
        n203 = Boolean To (0,1)(Boolean="Sweep\nContinuously") -> (0, 1=w399:i16)
        n204 = case shown="True" "Sweep\nContinuously" {
          tunnel: w394 -> [_ w402]
          tunnel: ["" ("String") w401] -> w395
          frame False {
          }
          frame True {
            n205 = case shown="True" w402 {
              tunnel: ["Sweeping Channel A" ("String") "Sweeping Channel B" ("String")] -> w401
              frame False {
              }
              frame True {
              }
            }
          }
        }
        "Swpc" <- w395
        n206 = Number To Decimal String(number=w399) -> (decimal integer string=w396:string)  [unwired: 1 in]
        n207 = Compound Arithmetic op=OR("Sweep\nContinuously", w390, w391, w392) -> (w393:bool)
        n208 = local write "Modon"(w393) -> ()
        n209 = Concatenate Strings("c" ("element"), w396, "g" ("element"), w396) -> (w388:string)
        n210 = call "LVSCharWrt.vi"("String In"=w388, "COM Port"=w387) -> ("ComError"=w386:bool)  [unwired: 9 in]
      }
      event "Sweep\nOnce": Value Change {
        # "Sweep Once"
        n211 = event-data() -> ()  [unwired: 1 in, 5 out]
        n212 = call "LVSCharWrt.vi"("String In"="g1" ("string"), "COM Port"=w406) -> ("ComError"=w405:bool)  [unwired: 9 in]
      }
      event "Continuous\nPM", "Dual Channel Mode": Value Change {
        # "Pulse Continuously"
        n213 = event-data() -> ()  [unwired: 1 in, 5 out]
        n214 = case shown="True" "Continuous\nPM" {
          tunnel: w420 -> [_ w428]
          tunnel: ["" ("String") w427] -> w421
          tunnel: "Dual Channel Mode" -> [_ w426]
          frame False {
          }
          frame True {
            n215 = case shown="True" w426 {
              tunnel: w428 -> [w430 w433]
              tunnel: [w429 w434] -> w427
              frame False {
                n216 = case shown="False" w430 {
                  tunnel: ["Modulating\nChannel A" ("String") "Modulating\nChannel B" ("String")] -> w429
                  frame False {
                  }
                  frame True {
                  }
                }
              }
              frame True {
                n217 = case shown="True" w433 {
                  tunnel: ["Modulating\nChannel A & B\n(A Controls)" ("String") "Modulating\nChannel A & B\n(B Controls)" ("String")] -> w434
                  frame False {
                  }
                  frame True {
                  }
                }
              }
            }
          }
        }
        "Pulsech" <- w421
        n218 = local read "Sweep\nContinuously"() -> (w416:bool)
        n219 = local read "Continuous AM"() -> (w417:bool)
        n220 = local read "Continuous FM"() -> (w418:bool)
        n221 = Boolean To (0,1)(Boolean="Continuous\nPM") -> (0, 1=w424:i16)
        n222 = Boolean To (0,1)(Boolean="Dual Channel Mode") -> (0, 1=w413:i16)
        n223 = Number To Decimal String(number=w424) -> (decimal integer string=w422:string)  [unwired: 1 in]
        n224 = Number To Decimal String(number=w413) -> (decimal integer string=w412:string)  [unwired: 1 in]
        n225 = Compound Arithmetic op=OR(w416, w417, w418, "Continuous\nPM") -> (w419:bool)
        n226 = Concatenate Strings("j" ("element"), w422, "D" ("element"), w412) -> (w410:string)
        n227 = local write "Modon"(w419) -> ()
        n228 = call "LVSCharWrt.vi"("String In"=w410, "COM Port"=w409) -> ("ComError"=w408:bool)  [unwired: 9 in]
      }
      event "Send Pulse\nBurst": Value Change {
        # "Send Pulse Burst"
        n229 = event-data() -> ()  [unwired: 1 in, 5 out]
        n230 = call "LVSCharWrt.vi"("String In"="G" ("write buffer"), "COM Port"=w439) -> ("ComError"=w437:bool)  [unwired: 9 in]
      }
      event "Continuous AM": Value Change {
        n231 = event-data() -> ()  [unwired: 1 in, 5 out]
        n232 = Boolean To (0,1)(Boolean="Continuous AM") -> (0, 1=w452:i16)
        n233 = local read "Sweep\nContinuously"() -> (w444:bool)
        n234 = local read "Continuous\nPM"() -> (w446:bool)
        n235 = Number To Decimal String(number=w452) -> (decimal integer string=w450:string)  [unwired: 1 in]
        n236 = local read "Continuous FM"() -> (w445:bool)
        n237 = case shown="True" "Continuous AM" {
          tunnel: w449 -> [_ w455]
          tunnel: ["" ("String") w454] -> w448
          frame False {
          }
          frame True {
            n238 = case shown="True" w455 {
              tunnel: ["Modulating\nChannel A" ("String") "Modulating\nChannel B" ("String")] -> w454
              frame False {
              }
              frame True {
              }
            }
          }
        }
        "AMch" <- w448
        n239 = Concatenate Strings("A" ("element"), w450) -> (w441:string)
        n240 = call "LVSCharWrt.vi"("String In"=w441, "COM Port"=w442) -> ("ComError"=w440:bool)  [unwired: 9 in]
        n241 = Compound Arithmetic op=OR(w444, "Continuous AM", w445, w446) -> (w447:bool)
        n242 = local write "Modon"(w447) -> ()
      }
      event "AM Freq (Hz)", "Minimum Power (dBm)", "Peak Power(dBm)", "Wave Shape", "Linear in?": Value Change {
        # "Setup Lookup Table for AM"
        n243 = event-data() -> ()  [unwired: 1 in, 5 out]
        n244 = local read "HD2"() -> (w458:bool)
        n245 = call "AMLUTwaveselHD2.vi"("AM Freq Hz"="AM Freq (Hz)", "Peak Power"="Peak Power(dBm)", "Min Power"="Minimum Power (dBm)", "Wave Shape"="Wave Shape", "HD2?"=w458, "Linear in?"="Linear in?") -> ("Waveform"=→"Waveform":dbl[], "Actual Freq"=→"Actual Freq (Hz)":dbl, "LUTsize"=→"Samples/Cycle":u8, "powerout"=w460:string)  [unwired: 6 in]
        n246 = call "LVSCharWrt.vi"("String In"=w460, "COM Port"=w461) -> ("ComError"=w459:bool)  [unwired: 9 in]
      }
      event "Save AM to ROM": Value Change {
        n247 = event-data() -> ()  [unwired: 1 in, 5 out]
        n248 = call "LVSCharWrt.vi"("String In"="@e" ("string"), "COM Port"=w471) -> ("ComError"=w470:bool)  [unwired: 9 in]
      }
      event "Read AM": Value Change {
        n249 = event-data() -> ()  [unwired: 1 in, 5 out]
        n250 = call "LVSgetAMtable.vi"("Serial Port Select"=w474) -> ("COM Error"=w473:bool, "Min dB"=w475:dbl, "Max dB"=w476:dbl, "Waveform Graph"=w477:dbl[], "AM Freq Hz"=w478:dbl)  [unwired: 5 in, 1 out]
        n251 = local write "Minimum Power (dBm)"(w475) -> ()
        n252 = local write "AM Freq (Hz)"(w478) -> ()
        n253 = local write "Waveform"(w477) -> ()
        n254 = local write "Peak Power(dBm)"(w476) -> ()
      }
      event "Save Settings\nto ROM": Value Change {
        n255 = event-data() -> ()  [unwired: 1 in, 5 out]
        n256 = call "LVSCharWrt.vi"("String In"="e" ("write buffer"), "COM Port"=w481) -> ("ComError"=w479:bool)  [unwired: 9 in]
      }
      event "Read\nVersion": Value Change {
        n257 = event-data() -> ()  [unwired: 1 in, 5 out]
        n258 = call "LVSWrt_Rd_Trm.vi"("WriteBuf"="v0" ("write buffer"), "COM Port"=w486) -> ("ComError"=w484:bool, "string read"=→"FW Version":string)  [unwired: 8 in]
        n259 = case shown="False" w484 {
          tunnel: w486 -> [w490 _]
          tunnel: [w487 TRUE] -> w482
          frame False {
            n260 = call "LVSWrt_Rd_Trm.vi"("WriteBuf"="v1" ("write buffer"), "COM Port"=w490) -> ("ComError"=w487:bool, "string read"=→"HW Version":string)  [unwired: 8 in]
          }
          frame True {
          }
        }
      }
      event "Get\nTemperature": Value Change {
        n261 = event-data() -> ()  [unwired: 1 in, 5 out]
        n262 = call "LVSWrt_Rd_Trm.vi"("WriteBuf"="z" ("write buffer"), "COM Port"=w495) -> ("ComError"=w492:bool, "string read"=→"Temperature":string)  [unwired: 8 in]
      }
      event "Reference (MHz)", "Reference Select": Value Change {
        n263 = event-data() -> ()  [unwired: 1 in, 5 out]
        n264 = Number To Decimal String(number="Reference Select") -> (decimal integer string=w502:string)  [unwired: 1 in]
        n265 = case shown="0, Default" "Reference Select" {
          tunnel: [w503 "*27.0" ("write buffer") "*10.0" ("write buffer")] -> w499
          frame 0, Default {
            n266 = Number To Fractional String(use system decimal point (T)=FALSE, number="Reference (MHz)") -> (F-format string=w507:string)  [unwired: 2 in]
            n267 = Concatenate Strings("*" ("write buffer"), w507) -> (w503:string)
            n268 = property on="Reference (MHz)" class="DigNum (strict)"("DisabledEnum"=T2."Enabled" ("Disabled")) -> ()  [unwired: 2 in, 2 out]
          }
          frame 1 {
            n269 = local write "Reference (MHz)"(27.0 ("Reference (MHz)")) -> ()
            n270 = property on="Reference (MHz)" class="DigNum (strict)"("DisabledEnum"=T2."Disabled and Grayed Out" ("Disabled")) -> ()  [unwired: 2 in, 2 out]
          }
          frame 2 {
            n271 = local write "Reference (MHz)"(10.0 ("Reference (MHz)")) -> ()
            n272 = property on="Reference (MHz)" class="DigNum (strict)"("DisabledEnum"=T2."Disabled and Grayed Out" ("Disabled")) -> ()  [unwired: 2 in, 2 out]
          }
        }
        n273 = Concatenate Strings("x" ("write buffer"), w502, w499) -> (w497:string)
        n274 = call "LVSCharWrt.vi"("String In"=w497, "COM Port"=w498) -> ("ComError"=w496:bool)  [unwired: 9 in]
      }
      event "PLL ICP": Value Change {
        n275 = event-data() -> ()  [unwired: 1 in, 5 out]
        n276 = Number To Decimal String(number="PLL ICP") -> (decimal integer string=w519:string)  [unwired: 1 in]
        n277 = Concatenate Strings("U" ("string"), w519) -> (w517:string)
        n278 = call "LVSCharWrt.vi"("String In"=w517, "COM Port"=w516) -> ("ComError"=w515:bool)  [unwired: 9 in]
      }
      event "MTLD": Value Change {
        n279 = event-data() -> ()  [unwired: 1 in, 5 out]
        n280 = Boolean To (0,1)(Boolean="MTLD") -> (0, 1=w525:i16)
        n281 = Number To Decimal String(number=w525) -> (decimal integer string=w526:string)  [unwired: 1 in]
        n282 = Concatenate Strings("d" ("string"), w526) -> (w522:string)
        n283 = call "LVSCharWrt.vi"("String In"=w522, "COM Port"=w523) -> ("ComError"=w521:bool)  [unwired: 9 in]
      }
      event "MUX Out Select": Value Change {
        n284 = event-data() -> ()  [unwired: 1 in, 5 out]
        n285 = Number To Decimal String(number="MUX Out Select") -> (decimal integer string=w532:string)  [unwired: 1 in]
        n286 = Concatenate Strings("m" ("string"), w532) -> (w529:string)
        n287 = call "LVSCharWrt.vi"("String In"=w529, "COM Port"=w530) -> ("ComError"=w528:bool)  [unwired: 9 in]
      }
      event "Channel\nSpacing": Value Change {
        n288 = event-data() -> ()  [unwired: 1 in, 6 out]
        n289 = Less?(x="Channel\nSpacing", y=100.0) -> (x < y?=w536:bool)
        n290 = Number To Fractional String(use system decimal point (T)=FALSE, number="Channel\nSpacing", precision (6)=i16 2) -> (F-format string=w545:string)  [unwired: 1 in]
        n291 = Not(x="CSD") -> (.not. x?=w534:bool)
        n292 = And(x=w536, y=w534) -> (x .and. y?=w537:bool)
        n293 = case shown="True" w537 {
          frame False {
          }
          frame True {
            n294 = local write "CSD"(TRUE ("CSD")) -> ()
            n295 = One Button Dialog(message="Phase tuning will be\nvery slow with settings\nbelow 100Hz Channel\nSpacing.  Especially\nat low RF frequencies.") -> ()  [unwired: 1 in, 1 out]
          }
        }
        n296 = Concatenate Strings("i" ("string"), w545) -> (w546:string)
        n297 = call "LVSCharWrt.vi"("String In"=w546, "COM Port"=w541) -> ("ComError"=w540:bool)  [unwired: 9 in]
      }
      event "Sync", "ChSt", "boot": Value Change {
        n298 = event-data() -> ()  [unwired: 1 in, 5 out]
        n299 = stacked-sequence {
          tunnel: w553 -> [w573 _]
          tunnel: w552 -> [_ _]
          tunnel: w551 -> [w563 _]
          tunnel: [w557 _] -> w550
          tunnel: [w554 _] -> w549
          frame #0 {
            # "Load settings from SynthHD"
            # "Only send one error."
            # "Scan for Devices"
            n300 = local read "COM Error"() -> (w576:bool)
            n301 = feedback #1() -> (w578:bool)  [unwired: 1 in]
            n302 = Equal?(x=w578, y=FALSE) -> (x = y?=w581:bool)
            n303 = feedback-in #1(w576) -> ()
            n304 = Equal?(x=w576, y=TRUE) -> (x = y?=w580:bool)
            n305 = And(x=w580, y=w581) -> (x .and. y?=w554:bool)
            n306 = Compound Arithmetic op=OR(w554, "Sync", "boot") -> (w575:bool)
            n307 = case shown="True" w575 {
              tunnel: [TRUE ("Prog Chan?") FALSE ("Prog Chan?")] -> w565
              tunnel: w563 -> [w681 _]
              tunnel: [w680 w686] -> w555
              frame False {
                n308 = case shown="False" w681 {
                  tunnel: ["B" ("Channel") "A" ("Channel")] -> w682
                  frame False {
                  }
                  frame True {
                  }
                }
                "Channel" <- w682
                n309 = local read "Serial Port Select"() -> (w680:refnum<visa-resource-name>)
              }
              frame True {
                n310 = call "LVSgetcomportSHD.vi"() -> ("Port"=w686:string, "Device"=→"Device Under Control":string)  [unwired: 9 in, 1 out]
                n311 = local write "Serial Port Select"(w686) -> ()
              }
            }
            n312 = call "LVSreadparams.vi"("Port In"=w555, "var query"=w573, "Get F&A"=TRUE, "Prog Chan?"=w565, "ChSt"=w563) -> ("RFonA"=w560:bool, "RFonB"=w559:bool, "LevA"=w561:bool, "LevB"=w562:bool, "FchA"=w572:dbl, "FchB"=w568:dbl, "ComError"=w557:bool, "AdBm"=w571:dbl, "BdBm"=w566:dbl, "NowLevel"=w570:bool, "cluster"=w558:T3, "NowFreq"=w564:dbl, "NowdBm"=w569:dbl)  [unwired: 8 in, 2 out]
            n313 = local write "Level A 2"(w561) -> ()
            n314 = local write "RFOnA2"(w560) -> ()
            n315 = local write "RF  FREQUENCY MHz A"(w572) -> ()
            n316 = local write "RF  FREQUENCY MHz"(w564) -> ()
            n317 = local write "POWER dBm A"(w571) -> ()
            n318 = local write "Level"(w570) -> ()
            n319 = local write "POWER dBm"(w569) -> ()
            n320 = local write "POWER dBm B"(w566) -> ()
            n321 = local write "RF  FREQUENCY MHz  B"(w568) -> ()
            n322 = local write "RFOnB2"(w559) -> ()
            n323 = local write "Level B 2"(w562) -> ()
            n324 = stacked-sequence {
              tunnel: w558 -> [w584 w613 w651 _ _]
              tunnel: w555 -> [_ _ w620 _ w663]
              frame #0 {
                n325 = Unbundle By Name(w584) -> ("[0]"=w589:dbl, "[2]"=w588:dbl, "[10]"=w583:dbl, "[30]"=w582:dbl)
                n326 = Equal To 0?(x=w589) -> (x = 0?=w585:bool)
                n327 = case shown="0, Default" w583 {
                  frame 0, Default {
                    n328 = property on="Reference (MHz)" class="DigNum (strict)"("DisabledEnum"=T2."Enabled" ("Disabled")) -> ()  [unwired: 2 in, 2 out]
                  }
                  frame 1 {
                    n329 = property on="Reference (MHz)" class="DigNum (strict)"("DisabledEnum"=T2."Disabled and Grayed Out" ("Disabled")) -> ()  [unwired: 2 in, 2 out]
                  }
                  frame 2 {
                    n330 = property on="Reference (MHz)" class="DigNum (strict)"("DisabledEnum"=T2."Disabled and Grayed Out" ("Disabled")) -> ()  [unwired: 2 in, 2 out]
                  }
                }
                n331 = local write "ChSt"(w585) -> ()
                n332 = case shown="True" w585 {
                  tunnel: ["B" ("Channel") "A" ("Channel")] -> w586
                  frame False {
                  }
                  frame True {
                  }
                }
                n333 = local write "Reference (MHz)"(w582) -> ()
                n334 = local write "Reference Select"(w583) -> ()
                n335 = Not Equal To 0?(x=w588) -> (x != 0?=w587:bool)
                n336 = local write "RF On"(w587) -> ()
                n337 = local write "Channel"(w586) -> ()
              }
              frame #1 {
                # "Sweep"
                n338 = Unbundle By Name(w613) -> ("[11]"=w604:dbl, "[12]"=w603:dbl, "[13]"=w612:dbl, "[14]"=w602:dbl, "[15]"=w600:dbl, "[16]"=w599:dbl, "[17]"=w611:dbl, "[18]"=w609:dbl, "[19]"=w608:dbl, "[20]"=w596:dbl, "[21]"=w601:dbl, "[22]"=w606:dbl)
                n339 = local read "SwType"() -> (w595:bool)
                n340 = Equal To 0?(x=w611) -> (x = 0?=w610:bool)
                n341 = Not Equal To 0?(x=w608) -> (x != 0?=w607:bool)
                n342 = Not Equal To 0?(x=w601) -> (x != 0?=w605:bool)
                n343 = case shown="0, Default" w596 {
                  tunnel: [w614 w616 TRUE ("SwType")] -> w598
                  tunnel: [enum32{"Linear", "List"}."Linear" ("Sweep") enum32{"Linear", "List"}."List" ("Sweep") enum32{"Linear", "List"}."Linear" ("Sweep")] -> w597
                  tunnel: w595 -> [w614 w616 _]
                  frame 0, Default {
                  }
                  frame 1 {
                  }
                  frame 2 {
                  }
                }
                n344 = local write "Step Size MHz (or %)"(w612) -> ()
                n345 = local write "Differential Freq"(w609) -> ()
                n346 = local write "sweepdiff"(w607) -> ()
                n347 = local write "Stop Frequency"(w603) -> ()
                n348 = local write "Start Frequency"(w604) -> ()
                n349 = local write "Start Amplitude"(w600) -> ()
                n350 = local write "Stop Amplitude"(w599) -> ()
                n351 = local write "Step Time (mS)"(w602) -> ()
                n352 = local write "sweepdir"(w610) -> ()
                n353 = local write "Sweep\nContinuously"(w605) -> ()
                n354 = local write "Trigger"(w606) -> ()
                n355 = property on="Sweep" class="TabCtl (strict)"("Value"=w597) -> ()  [unwired: 2 in, 2 out]
                n356 = local write "SwType"(w598) -> ()
              }
              frame #2 {
                # "Mods"
                n357 = Unbundle By Name(w651) -> ("[25]"=w648:dbl, "[26]"=w647:dbl, "[27]"=w646:dbl, "[28]"=w645:dbl, "[29]"=w644:dbl, "[31]"=w643:dbl, "[32]"=w642:dbl, "[33]"=w640:dbl, "[34]"=w639:dbl, "[35]"=w637:dbl, "[36]"=w636:dbl, "[37]"=w634:dbl, "[38]"=w632:dbl, "[39]"=w631:dbl, "[40]"=w630:dbl, "[41]"=w628:dbl, "[42]"=w627:dbl, "[43]"=w625:dbl)  [unwired: 2 out]
                n358 = call "LVSgetAMtable.vi"("Serial Port Select"=w620) -> ("Min dB"=w621:dbl, "Max dB"=w622:dbl, "Waveform Graph"=w623:dbl[], "AM Freq Hz"=w624:dbl)  [unwired: 5 in, 2 out]
                n359 = Not Equal To 0?(x=w637) -> (x != 0?=w638:bool)
                n360 = Not Equal To 0?(x=w634) -> (x != 0?=w635:bool)
                n361 = Not Equal To 0?(x=w631) -> (x != 0?=w633:bool)
                n362 = Not Equal To 0?(x=w644) -> (x != 0?=w649:bool)
                n363 = Not Equal To 0?(x=w628) -> (x != 0?=w629:bool)
                n364 = Not Equal To 0?(x=w648) -> (x != 0?=w650:bool)
                n365 = Not Equal To 0?(x=w639) -> (x != 0?=w641:bool)
                n366 = local write "Fundamental\nFeedback Mode"(w638) -> ()
                n367 = local write "FM Deviation (+/- Hz)"(w642) -> ()
                n368 = local write "FM Function"(w636) -> ()
                n369 = local write "Invert\nPulse"(w635) -> ()
                n370 = local write "MTLD"(w633) -> ()
                n371 = local write "Minimum Power (dBm)"(w621) -> ()
                n372 = local write "PLL ICP"(w632) -> ()
                n373 = local write "AM Freq (Hz)"(w624) -> ()
                n374 = local write "# of Pulses in Burst"(w645) -> ()
                n375 = local write "Waveform"(w623) -> ()
                n376 = local write "Peak Power(dBm)"(w622) -> ()
                n377 = local write "Continuous\nPM"(w649) -> ()
                n378 = local write "FM Rate (Hz)"(w643) -> ()
                n379 = local write "MUX Out Select"(w630) -> ()
                n380 = local write "On Time (uS)"(w647) -> ()
                n381 = local write "Off Time (uS)"(w646) -> ()
                n382 = local write "FM Samples in Burst"(w640) -> ()
                n383 = local write "Continuous AM"(w650) -> ()
                n384 = Not Equal To 0?(x=w625) -> (x != 0?=w626:bool)
                n385 = local write "Dual Channel Mode"(w629) -> ()
                n386 = local write "Continuous FM"(w641) -> ()
                n387 = local write "AutoCal"(w626) -> ()
                n388 = local write "PHASE Degrees"(w627) -> ()
              }
              frame #3 {
                n389 = local read "Sweep\nContinuously"() -> (w653:bool)
                n390 = local read "Continuous AM"() -> (w654:bool)
                n391 = local read "Continuous\nPM"() -> (w656:bool)
                n392 = local read "Continuous FM"() -> (w655:bool)
                n393 = Compound Arithmetic op=OR(w653, w654, w655, w656) -> (w657:bool)
                n394 = local write "boot"(FALSE ("boot")) -> ()
                n395 = local write "Modon"(w657) -> ()
              }
              frame #4 {
                # "2019 ver responds\nwith HDPRO or\nHD"
                n396 = call "LVSWrt_Rd_Trm.vi"("WriteBuf"="v2" ("String In"), "COM Port"=w663) -> ("string read"=w660:string)  [unwired: 8 in, 1 out]
                n397 = Equal?(x=w660, y="HD\n") -> (x = y?=w661:bool)
                n398 = Equal?(x=w660, y="HDPRO\n") -> (x = y?=w659:bool)
                n399 = Or(x=w661, y=w659) -> (x .or. y?=w658:bool)
                "HD2" <- w658
                n400 = case shown="False" w658 {
                  tunnel: w663 -> [_ w670]
                  tunnel: w659 -> [_ w669]
                  frame False {
                    w666 = 53.0 ("Data Entry Limits:Minimum")
                    w667 = 13999.999 ("Data Entry Limits:Maximum")
                    # "v1 HD and Pro"
                    n401 = property on="Fundamental\nFeedback Mode" class="Bool (strict)"("Strings [4]"=string[] ["Feedback Mode\nis Divided", "Feedback Mode\nis Fundamental"]) -> ()  [unwired: 2 in, 2 out]
                    n402 = property on="RF  FREQUENCY MHz" class="DigNum (strict)"("Maximum"=w667) -> ()  [unwired: 2 in, 2 out]
                    n403 = property on="Start Frequency" class="DigNum (strict)"("Maximum"=w667) -> ()  [unwired: 2 in, 2 out]
                    n404 = property on="RF  FREQUENCY MHz" class="DigNum (strict)"("Minimum"=w666) -> ()  [unwired: 2 in, 2 out]
                    n405 = property on="Stop Frequency" class="DigNum (strict)"("Maximum"=w667) -> ()  [unwired: 2 in, 2 out]
                    n406 = property on="Start Frequency" class="DigNum (strict)"("Minimum"=w666) -> ()  [unwired: 2 in, 2 out]
                    n407 = property on="Stop Frequency" class="DigNum (strict)"("Minimum"=w666) -> ()  [unwired: 2 in, 2 out]
                  }
                  frame True {
                    n408 = stacked-sequence {
                      tunnel: w670 -> [w677]
                      frame #0 {
                        n409 = call "LVSWrt_Rd_Trm.vi"("WriteBuf"="i?" ("String In"), "COM Port"=w677) -> ("string read"=w676:string)  [unwired: 8 in, 1 out]
                        n410 = Fract/Exp String To Number(string=w676) -> (number=w675:dbl)  [unwired: 3 in, 1 out]
                        n411 = local write "Channel\nSpacing"(w675) -> ()
                        n412 = property on="Fundamental\nFeedback Mode" class="Bool (strict)"("Strings [4]"=string[] ["Reference\nX2 OFF", "Reference\nX2 ON"]) -> ()  [unwired: 2 in, 2 out]
                      }
                    }
                    n413 = case shown="True" w669 {
                      frame False {
                        w671 = 10.0 ("Data Entry Limits:Minimum")
                        w672 = 15000.0 ("Data Entry Limits:Maximum")
                        # "HD 2"
                        n414 = property on="RF  FREQUENCY MHz" class="DigNum (strict)"("Maximum"=w672) -> ()  [unwired: 2 in, 2 out]
                        n415 = property on="Start Frequency" class="DigNum (strict)"("Maximum"=w672) -> ()  [unwired: 2 in, 2 out]
                        n416 = property on="RF  FREQUENCY MHz" class="DigNum (strict)"("Minimum"=w671) -> ()  [unwired: 2 in, 2 out]
                        n417 = property on="Stop Frequency" class="DigNum (strict)"("Maximum"=w672) -> ()  [unwired: 2 in, 2 out]
                        n418 = property on="Start Frequency" class="DigNum (strict)"("Minimum"=w671) -> ()  [unwired: 2 in, 2 out]
                        n419 = property on="Stop Frequency" class="DigNum (strict)"("Minimum"=w671) -> ()  [unwired: 2 in, 2 out]
                      }
                      frame True {
                        w673 = 10.0 ("Data Entry Limits:Minimum")
                        w674 = 24000.0 ("Data Entry Limits:Maximum")
                        # "HDPRO 2"
                        n420 = property on="RF  FREQUENCY MHz" class="DigNum (strict)"("Maximum"=w674) -> ()  [unwired: 2 in, 2 out]
                        n421 = property on="Start Frequency" class="DigNum (strict)"("Maximum"=w674) -> ()  [unwired: 2 in, 2 out]
                        n422 = property on="RF  FREQUENCY MHz" class="DigNum (strict)"("Minimum"=w673) -> ()  [unwired: 2 in, 2 out]
                        n423 = property on="Stop Frequency" class="DigNum (strict)"("Maximum"=w674) -> ()  [unwired: 2 in, 2 out]
                        n424 = property on="Start Frequency" class="DigNum (strict)"("Minimum"=w673) -> ()  [unwired: 2 in, 2 out]
                        n425 = property on="Stop Frequency" class="DigNum (strict)"("Minimum"=w673) -> ()  [unwired: 2 in, 2 out]
                      }
                    }
                  }
                }
              }
            }
          }
          frame #1 {
            w689 = TRUE ("Reset")
            # "reset knob memory between channels"
            # "Keep knobs working nice by\nloading with other channel value"
            n426 = flat-sequence {
              tunnel: [w696] -> w691
              tunnel: w691 -> [w698]
              tunnel: [w697] -> w690
              tunnel: w690 -> [w700]
              frame #0 {
                n427 = local read "Powerkn"() -> (w696:i8)
              }
              frame #1 {
                n428 = feedback #2(i8 1 ("Freqkn")) -> (w697:i8)
                n429 = feedback-in #2(w698) -> ()
              }
              frame #2 {
                n430 = local write "Powerkn"(w700) -> ()
              }
            }
            n431 = flat-sequence {
              tunnel: [w706] -> w695
              tunnel: w695 -> [w708]
              tunnel: [w707] -> w694
              tunnel: w694 -> [w710]
              frame #0 {
                n432 = local read "Freqkn"() -> (w706:i8)
              }
              frame #1 {
                n433 = feedback #3(i8 1 ("Freqkn")) -> (w707:i8)
                n434 = feedback-in #3(w708) -> ()
              }
              frame #2 {
                n435 = local write "Freqkn"(w710) -> ()
              }
            }
            n436 = flat-sequence {
              tunnel: [w701] -> w693
              tunnel: w693 -> [w703]
              tunnel: [w702] -> w692
              tunnel: w692 -> [w705]
              frame #0 {
                n437 = local read "Phasekn"() -> (w701:i8)
              }
              frame #1 {
                n438 = feedback #4(i8 1 ("Freqkn")) -> (w702:i8)
                n439 = feedback-in #4(w703) -> ()
              }
              frame #2 {
                n440 = local write "Phasekn"(w705) -> ()
              }
            }
            n441 = local write "FKNR"(w689) -> ()
            n442 = local write "PKNR"(w689) -> ()
            n443 = local write "AKNR"(w689) -> ()
          }
        }
      }
      event "Modon": Value Change {
        n444 = event-data() -> ()  [unwired: 1 in, 5 out]
        n445 = case shown="True" "Modon" {
          tunnel: w712 -> [w715 _]
          tunnel: [w714 w718] -> w711
          frame False {
            w717 = FALSE ("Sweep\nContinuously")
            # "Turn off all mods"
            n446 = call "LVSCharWrt.vi"("String In"="g0c0/0j0A0" ("string"), "COM Port"=w715) -> ("ComError"=w714:bool)  [unwired: 9 in]
            n447 = local write "Sweep\nContinuously"(w717) -> ()
            n448 = local write "Continuous AM"(w717) -> ()
            n449 = local write "Continuous\nPM"(w717) -> ()
            n450 = local write "Continuous FM"(w717) -> ()
          }
          frame True {
            w718 = FALSE ("Modon")
            n451 = local write "Modon"(w718) -> ()
          }
        }
      }
      event "FM Rate (Hz)", "FM Deviation (+/- Hz)", "FM Samples in Burst", "FM Function": Value Change {
        w731 = 16.0 ("y")
        n452 = event-data() -> ()  [unwired: 1 in, 5 out]
        n453 = Divide(x=u16 464 ("y"), y="FM Rate (Hz)") -> (x/y=w734:dbl)
        n454 = Number To Decimal String(number="FM Function") -> (decimal integer string=w737:string)  [unwired: 1 in]
        n455 = Number To Decimal String(number="FM Deviation (+/- Hz)") -> (decimal integer string=w742:string)  [unwired: 1 in]
        n456 = Number To Decimal String(number="FM Samples in Burst") -> (decimal integer string=w739:string)  [unwired: 1 in]
        n457 = Number To Decimal String(number="FM Rate (Hz)") -> (decimal integer string=w745:string)  [unwired: 1 in]
        n458 = Round Toward -Infinity(1:w734) -> (0:w733:dbl)
        n459 = Multiply(x=w733, y=w731) -> (x*y=w732:dbl)
        n460 = Add(x=w732, y=w731) -> (x+y=w730:dbl)
        n461 = Multiply(x="FM Rate (Hz)", y=w730) -> (x*y=w728:dbl)
        n462 = Concatenate Strings("<" ("string"), w745, ">" ("string"), w742, "," ("string"), w739, ";" ("string"), w737) -> (w721:string)
        n463 = Divide(x=1000000.0, y=w728) -> (x/y=w726:dbl)
        n464 = Round Toward -Infinity(1:w726) -> (0:w725:dbl)
        n465 = call "LVSCharWrt.vi"("String In"=w721, "COM Port"=w720) -> ("ComError"=w719:bool)  [unwired: 9 in]
        n466 = In Range and Coerce(upper limit=100.0, x=w725, lower limit=0.0) -> (coerced(x)=→"FM Samples / Cycle":dbl)  [unwired: 1 out]
      }
      event "Continuous FM": Value Change {
        n467 = event-data() -> ()  [unwired: 1 in, 5 out]
        n468 = Boolean To (0,1)(Boolean="Continuous FM") -> (0, 1=w758:i16)
        n469 = Number To Decimal String(number=w758) -> (decimal integer string=w757:string)  [unwired: 1 in]
        n470 = case shown="True" "Continuous FM" {
          tunnel: w752 -> [_ w762]
          tunnel: ["" ("String") w761] -> w750
          frame False {
          }
          frame True {
            n471 = case shown="True" w762 {
              tunnel: ["Modulating\nChannel A" ("String") "Modulating\nChannel B" ("String")] -> w761
              frame False {
              }
              frame True {
              }
            }
          }
        }
        "FMch" <- w750
        n472 = local read "Sweep\nContinuously"() -> (w753:bool)
        n473 = local read "Continuous AM"() -> (w754:bool)
        n474 = local read "Continuous\nPM"() -> (w755:bool)
        n475 = Concatenate Strings("/" ("string"), w757) -> (w749:string)
        n476 = call "LVSCharWrt.vi"("String In"=w749, "COM Port"=w748) -> ("ComError"=w747:bool)  [unwired: 9 in]
        n477 = Compound Arithmetic op=OR(w753, w754, "Continuous FM", w755) -> (w756:bool)
        n478 = local write "Modon"(w756) -> ()
      }
      event "Query1", "Query2", "Query3", "Query4": Value Change {
        n479 = event-data() -> ()  [unwired: 1 in, 6 out]
        n480 = case shown="True" "Query1" {
          tunnel: ["" ("write buffer") "?" ("write buffer")] -> w775
          frame False {
          }
          frame True {
          }
        }
        n481 = case shown="True" "Query2" {
          tunnel: ["" ("write buffer") "HV" ("write buffer")] -> w772
          frame False {
          }
          frame True {
          }
        }
        n482 = case shown="True" "Query3" {
          tunnel: ["" ("write buffer") "H?" ("write buffer")] -> w771
          frame False {
          }
          frame True {
          }
        }
        n483 = case shown="True" "Query4" {
          tunnel: ["" ("write buffer") "HA" ("write buffer")] -> w769
          frame False {
          }
          frame True {
          }
        }
        n484 = Concatenate Strings(w775, w772, w771, w769) -> (w768:string)
        n485 = call "LVSPrtHlpHD.vi"("Help?"=w768, "VISA resource name"=w766) -> ("error?"=w765:bool, "string read"=→"read buffer":string)  [unwired: 8 in]
      }
      event Mouse Wheel {
        n486 = event-data() -> ("Coords"=w788:T4, "Delta"=w787:i32)  [unwired: 1 in, 8 out]
        n487 = local read "Main Tab"() -> (w786:T1)
        n488 = case shown="\"Generator\"" w786 {
          tunnel: w788 -> [w808 _]
          tunnel: w787 -> [w790 _]
          frame "Generator" {
            n489 = Unbundle By Name(w808) -> ("Vertical"=w793:i32, "Horizontal"=w794:i32)
            n490 = Greater?(x=w793, y=0) -> (0:w810:bool)
            n491 = Less?(x=w793, y=137) -> (x < y?=w809:bool)
            n492 = Greater?(x=w794, y=334) -> (0:w797:bool)
            n493 = Greater?(x=w794, y=0) -> (0:w805:bool)
            n494 = Greater?(x=w794, y=164) -> (0:w801:bool)
            n495 = Less?(x=w794, y=484) -> (x < y?=w796:bool)
            n496 = Less?(x=w794, y=153) -> (x < y?=w804:bool)
            n497 = Less?(x=w794, y=323) -> (x < y?=w800:bool)
            n498 = And(x=w810, y=w809) -> (x .and. y?=w795:bool)
            n499 = Compound Arithmetic op=AND(w795, w797, w796) -> (w789:bool)
            n500 = Compound Arithmetic op=AND(w795, w801, w800) -> (w791:bool)
            n501 = Compound Arithmetic op=AND(w795, w805, w804) -> (w792:bool)
            n502 = case shown="True" w792 {
              tunnel: w790 -> [_ w847]
              frame False {
              }
              frame True {
                n503 = local read "Freqkn"() -> (w842:i8)
                n504 = Add(x=w842, y=w847) -> (x+y=w844:i32)
                n505 = Greater?(x=w842, y=i8 19) -> (0:w845:bool)
                n506 = Less?(x=w842, y=i8 1) -> (x < y?=w840:bool)
                n507 = case shown="True" w845 {
                  tunnel: w844 -> [w850 _]
                  tunnel: [w850 i8 1 ("Freqkn")] -> w843
                  frame False {
                  }
                  frame True {
                  }
                }
                n508 = case shown="True" w840 {
                  tunnel: w843 -> [w848 _]
                  tunnel: [w848 i8 19 ("Freqkn")] -> w839
                  frame False {
                  }
                  frame True {
                  }
                }
                n509 = property on="Freqkn" class="Knob (strict)"("Val(Sgnl)"=w839) -> ()  [unwired: 2 in, 2 out]
              }
            }
            n510 = case shown="True" w791 {
              tunnel: w790 -> [_ w834]
              frame False {
              }
              frame True {
                n511 = local read "Phasekn"() -> (w827:i8)
                n512 = Add(x=w827, y=w834) -> (x+y=w831:i32)
                n513 = Greater?(x=w827, y=i8 19) -> (0:w832:bool)
                n514 = Less?(x=w827, y=i8 1) -> (x < y?=w828:bool)
                n515 = case shown="True" w832 {
                  tunnel: w831 -> [w837 _]
                  tunnel: [w837 i8 1 ("Freqkn")] -> w830
                  frame False {
                  }
                  frame True {
                  }
                }
                n516 = case shown="True" w828 {
                  tunnel: w830 -> [w835 _]
                  tunnel: [w835 i8 19 ("Freqkn")] -> w826
                  frame False {
                  }
                  frame True {
                  }
                }
                n517 = property on="Phasekn" class="Knob (strict)"("Val(Sgnl)"=w826) -> ()  [unwired: 2 in, 2 out]
              }
            }
            n518 = case shown="True" w789 {
              tunnel: w790 -> [_ w821]
              frame False {
              }
              frame True {
                n519 = local read "Powerkn"() -> (w814:i8)
                n520 = Add(x=w814, y=w821) -> (x+y=w818:i32)
                n521 = Greater?(x=w814, y=i8 19) -> (0:w819:bool)
                n522 = Less?(x=w814, y=i8 1) -> (x < y?=w815:bool)
                n523 = case shown="True" w819 {
                  tunnel: w818 -> [w824 _]
                  tunnel: [w824 i8 1 ("Freqkn")] -> w817
                  frame False {
                  }
                  frame True {
                  }
                }
                n524 = case shown="True" w815 {
                  tunnel: w817 -> [w822 _]
                  tunnel: [w822 i8 19 ("Freqkn")] -> w813
                  frame False {
                  }
                  frame True {
                  }
                }
                n525 = property on="Powerkn" class="Knob (strict)"("Val(Sgnl)"=w813) -> ()  [unwired: 2 in, 2 out]
              }
            }
          }
          frame "Sweep", Default {
          }
        }
        n526 = local read "COM Error"() -> (w785:bool)
      }
      event "stop": Value Change {
        n527 = event-data() -> ()  [unwired: 1 in, 5 out]
      }
      event Panel Close? {
        w854 = TRUE ("Discard?")
        n528 = event-data() -> ("VIRef"=w855:refnum<vi>)  [unwired: 1 in]
        n529 = Close Reference(reference=w855) -> ()  [unwired: 1 in, 1 out]
        n530 = event-data("Discard?"=w854) -> ()  [unwired: 1 in, 1 out]
      }
      event Timeout {
        n531 = event-data() -> ()  [unwired: 1 in, 2 out]
      }
      event "Get Phase\nLock Status": Value Change {
        n532 = event-data() -> ()  [unwired: 1 in, 5 out]
        n533 = case shown="True" "Get Phase\nLock Status" {
          tunnel: [w860 w867] -> w859
          tunnel: w858 -> [_ w864]
          tunnel: [w860 w861] -> w857
          frame False {
            w860 = FALSE
          }
          frame True {
            n534 = call "LVSWrt_Rd_Trm.vi"("WriteBuf"="p" ("write buffer"), "COM Port"=w864) -> ("ComError"=w861:bool, "string read"=w862:string)  [unwired: 8 in]
            n535 = Fract/Exp String To Number(string=w862) -> (number=w866:dbl)  [unwired: 3 in, 1 out]
            n536 = Not Equal?(x=0.0, y=w866) -> (x != y?=w867:bool)
          }
        }
        "Lock" <- w859
      }
      event "Re-Init Settings\nto Default": Value Change {
        n537 = event-data() -> ()  [unwired: 1 in, 5 out]
        n538 = call "LVSWrt_Rd_Trm.vi"("WriteBuf"="v" ("write buffer"), "COM Port"=w870) -> ("string read"=w868:string)  [unwired: 8 in, 1 out]
        n539 = String Subset(string=w868, offset (0)=17, length (rest)=1 ("length (rest)")) -> (substring=w874:string)
        n540 = Decimal String To Number(string=w874) -> (number=w873:i32)  [unwired: 2 in, 1 out]
        n541 = Greater?(x=w873, y=1) -> (0:w871:bool)
        n542 = case shown="True" w871 {
          tunnel: w870 -> [w877 w888]
          frame False {
            n543 = stacked-sequence {
              tunnel: w877 -> [w878 _ _ w882]
              frame #0 {
                # "Re-init firmware"
                n544 = call "LVSCharWrt.vi"("String In"="|w" ("write buffer"), "COM Port"=w878) -> ()  [unwired: 9 in, 1 out]
              }
              frame #1 {
                # "wait for firmware reboot"
                n545 = Wait (ms)(milliseconds to wait=u32 2000) -> ()  [unwired: 1 out]
              }
              frame #2 {
                n546 = One Button Dialog(message="Re-init complete.  Please\nclick Scan Devices.") -> ()  [unwired: 1 in, 1 out]
              }
              frame #3 {
                # "update this for turning off mods and setting temp comp"
                # "Program factory\ndefaults"
                n547 = call "createtable.vi"() -> ("tab output"=w885:string)  [unwired: 11 in]
                n548 = call "AMLUTwaveselHD2.vi"() -> ("powerout"=w886:string)  [unwired: 12 in, 3 out]
                n549 = Concatenate Strings(w886, "@e" ("string"), w885, "x1*27.0C1g0c0G0j0A0/0E0r0Z3f1000.0W0.0C0g0c0G0j0A0/0E1r1Z3f1000.0W0.0e" ("write buffer")) -> (w883:string)
                n550 = call "LVSCharWrt.vi"("String In"=w883, "COM Port"=w882) -> ()  [unwired: 9 in, 1 out]
              }
            }
          }
          frame True {
            # "reset command is |1812|z"
            n551 = stacked-sequence {
              tunnel: w888 -> [w889 _ _]
              frame #0 {
                n552 = call "LVSCharWrt.vi"("String In"="|1812|z" ("write buffer"), "COM Port"=w889) -> ()  [unwired: 9 in, 1 out]
              }
              frame #1 {
                # "wait for firmware reboot"
                n553 = Wait (ms)(milliseconds to wait=u32 2000) -> ()  [unwired: 1 out]
              }
              frame #2 {
                n554 = One Button Dialog(message="Re-init complete.  Please\nclick Scan Devices.") -> ()  [unwired: 1 in, 1 out]
              }
            }
          }
        }
      }
    }
    "COM Error" <- w15
    n555 = Not(x=w12) -> (.not. x?=w11:bool)
    n556 = feedback #5(w11) -> (w20:bool)
    n557 = feedback-in #5(w15) -> ()
    n558 = Equal?(x=w20, y=FALSE) -> (x = y?=w18:bool)
    n559 = Equal?(x=w15, y=TRUE) -> (x = y?=w19:bool)
    n560 = And(x=w19, y=w18) -> (x .and. y?=w13:bool)
    n561 = case shown="True" w13 {
      tunnel: "SynthHD Not Detected\nPlease Connect and Rescan" ("message") -> [_ w32]
      frame False {
      }
      frame True {
        n562 = Two Button Dialog(message=w32) -> ()  [unwired: 2 in, 1 out]
      }
    }
  }
  n563 = case shown="False" w5 {
    frame False {
      n564 = Open VI Reference(vi path=path "SynthHD_3_2a.vi") -> (vi reference=w894:refnum<vi>)  [unwired: 5 in, 1 out]
      n565 = invoke class="VI" method="FP.Close"(reference=w894) -> ()  [unwired: 2 in, 3 out]
    }
    frame True {
    }
  }
